vi "MegaAwesome_9_21_12b_JW.vi"() -> ()   [LabVIEW 2011]
uses:
  MegaAwesome_States.ctl
  <vilib>/Utility/inputDevices.llb/keyboardAcquire.vi
  <vilib>/Utility/file.llb/Read From Spreadsheet File (string).vi
  <vilib>/Utility/file.llb/Write To Spreadsheet File (string).vi
panel:
  out "ROI Descriptor out":T1 {"Contours"."Type" items=["No Selection", "Point", "Line", "Rectangle", "Oval", "Polygon", "Freehand Region", "Annulus", "Unused2", "Unused3", "Broken Line", "Freehand Line", "Rotated Rectangle"]}
  out "ROI Descriptor":T1 {"Contours"."Type" items=["No Selection", "Point", "Line", "Rectangle", "Oval", "Polygon", "Freehand Region", "Annulus", "Unused2", "Unused3", "Broken Line", "Freehand Line", "Rotated Rectangle"]}
  in  "Slider Min":dbl=5.0
  in  "Slider Max":dbl=5.0
  out "Opj X Axis":string
  out "X Axis Display Type":string
  in  "Index-Sat":dbl=5.0
  in  "Index-Lin":dbl=5.0
  in  "IndexLog-Lin":dbl=5.0
  in  "IndexLog-Sat":dbl=5.0 caption="Num Pts"
  out "Lin Id-Log Used":dbl[](array[numeric])
  out "Lin-Vg Array-Log Used":dbl[](array[numeric])
  in  "New: Comments":string
  out "Save Array":string[][](array[string])
  out "Folder Index":i32 caption="Length"
  out "Sat Id-Used":dbl[](array[numeric])
  out "Sat Vg Array-Used":dbl[](array[numeric])
  out "Vg Array-Log-Used":dbl[](array[numeric])
  out "Sat Id-Log-Used":dbl[](array[numeric])
  out "Lin Id-Used":dbl[](array[numeric])
  out "Lin-Vg Array-Used":dbl[](array[numeric])
  out "Lin Vd":dbl
  out "Recorded Prop":T2
  out "Current State":T3
  in  "Main Tab Control":T4(tab)
  in  "1) Transport":bool caption="2) Transport"
  in  "Image Analysis":bool caption="1) Image Analysis"
  in  "Transport\nFolder":path caption="Transport Folder"
  out "Transport\nFile":path=path "D:/UserData/Desktop/Jeremy/WFU/Research/Programs/VI mods/Image Not Found.png" caption="Transport File"
  in  "Image Folder":path
  out "Image File":path=path "D:/UserData/Desktop/Jeremy/WFU/Research/Programs/VI mods/Image Not Found.png"
  in  "Transfer File":path
  out "Transfer Folder":path
  out "Fabrication Prop":T5
  out "Distances":dbl[](array[numeric])
  in  "Zoom":i16(slide)=-3 scale=-5.0..5.0
  in  "Magnification":u16(ring) items=["5x", "10x", "20x", "50x", "80x"]
  in  "Undo Button":bool
  in  "Remove Button":bool
  in  "Transfer Plots":T6(tab)=enum."Saturation"
  in  "Lin-Trans Slider":dbl(slide) step=1.0 scale=-40.0..40.0 scale format="%#_1p"
  out "Sqrt-Lin":cluster{dbl[], dbl[]}[](graph)
  in  "Sat-Trans Slider":dbl(slide) step=1.0 scale=-40.0..40.0 scale format="%#_1p"
  out "Sqrt-Sat":cluster{dbl[], dbl[]}[](graph)
  out "Raw- Lin":cluster{dbl[], dbl[]}[](graph)
  out "Raw- Sat":cluster{dbl[], dbl[]}[](graph)
  in  "Log Plots":enum32{"Linear", "Saturation", "Transport"}(tab)=enum."Saturation"
  in  "Lin-Log Slider":dbl(slide) step=1.0 scale=-40.0..40.0 scale format="%#_1p"
  out "Log-Lin":cluster{dbl[], dbl[]}[](graph)
  in  "Sat-Log Slider":dbl(slide) step=1.0 scale=-40.0..40.0 scale format="%#_1p"
  out "Sat-Log":cluster{dbl[], dbl[]}[](graph)
  out "Transport":cluster{dbl[], dbl[]}[](graph)
  in  "Manual Controls":T7
  in  "File Controls":T8
  out "Date Recorded":string="Date Recorded" caption="Measured"
  out "Data Name:":string
  out "Image Name":string
  out "Index":string
  out "Date Created":string caption="Fabricated"
  in  "Comments:":string
  out "Rec: Length":dbl caption="Length" format="%#_3g"
  out "Rec: Width":dbl caption="Width" format="%#_4g"
  out "Rec: Dielectric (d)":dbl caption="Dielectric (d)" format="%#_3g"
  in  "New: Dielectric":dbl
  in  "New: Length":dbl
  in  "New: Width":dbl
  out "Rec: Temp":dbl caption="Sample Temp" format="%.1f"
  in  "New: Temp":dbl format="%.1f"
  out "Image Out":T9(plugin-control)
  in  "Num Pts":dbl=5.0
  in  "Num Pts Log":dbl=5.0 caption="Num Pts"
  out "Recorded Values Cluster":T10
  out "Calculated Values Cluster":T10 caption="Recorded Values Cluster"
  out "Re-Calculated Values Cluster":T10 caption="Recorded Values Cluster"
  in  "Independant Variable:":string(combo)="Length (um):"
  out "Image Preview":T9(plugin-control)
  out "Total Width":dbl
  in  "Room Temp":dbl=294.0
  in  "No Image\n File":path=path "\\\\acad1\\physics/Jurchescu-group/JW-PD/Mega Awesome/Image Not Found.png" caption="No Image File"
  in  "Origin Project File":path=path "\\\\acad1\\physics/Jurchescu-group/JW-PD/Group Library/Origin Project Files/DeviceData_8_10_12a_JW.opj"
  in  "No Transport\n File":path=path "\\\\acad1\\physics/Jurchescu-group/JW-PD/Mega Awesome/Image Not Found.png" caption="No Transport File"
  in  "Transport Style Controls":T11={"Transport Line Size"=1, "Transport Line Color"=16772608} {"Transport Line Size" items=["Extra Small", "Small", "Medium", "Large", "Extra Large"]}
  # "Transfer Location"
  # "What else would you like to view during your analysis?"
  # "Image Location"
  # "Transport Location"
  # "Recorded"
  # "Calculated"
  # "Re-Calculated"
  # "Manual"
  # "Used points display at y=0\nValues are wrong w/ slider"
  # "Slider\nDoesn't\nWork"
  # "Slider\nDoesn't\nWork"
  # "No new points displayed"
  # "Default File Choices"
  # "Default Analysis Values"
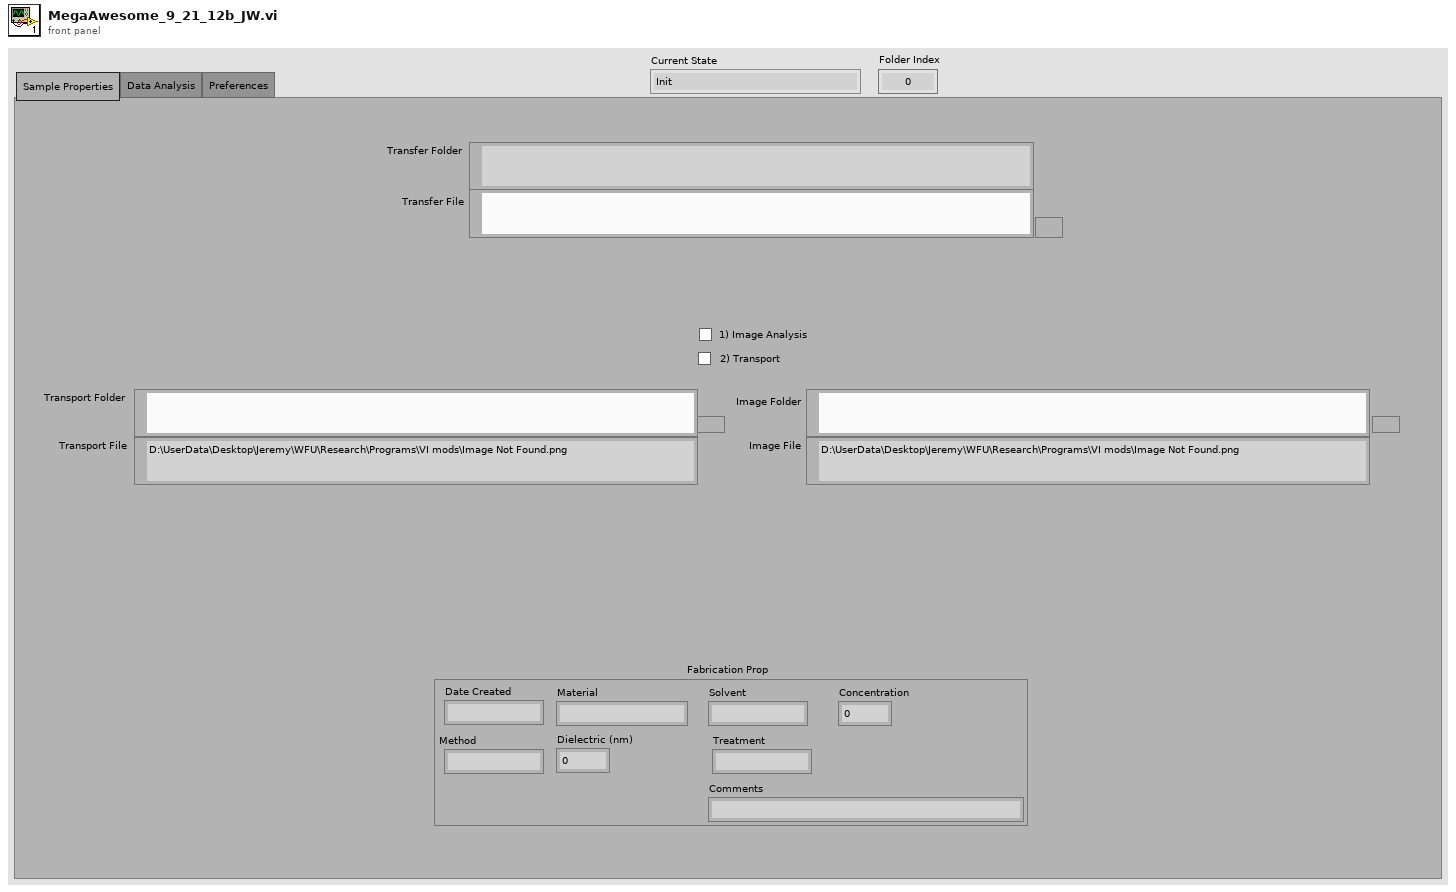
[diagram p1: front panel]
types:
  T1 = typedef "ROI Descriptor" = cluster{"Global Rectangle":i32[], "Contours":cluster{"ID":enum32{"External", "Internal"}, "Type":u32, "Coordinates":i32[]}[]}
  T2 = cluster{"Date Recorded":string, "Index":string, "Length":dbl, "Width":dbl, "Sample Temp":dbl}
  T3 = typedef "MegaAwesome_States.ctl" = enum16{"Init", "File Missing", "No Event", "Read Data", "Calculated Values", "Re-Calculated Values", "Next File", "Previous File", "Discard File", "Save", "Save Lines", "Export", "Exit"}
  T4 = enum32{"Sample Properties", "Data Analysis", "Preferences"}
  T5 = cluster{"Date Created":string, "Material":string, "Solvent":string, "Concentration":dbl, "Method":string, "Dielectric (nm)":dbl, "Treatment":string, "Comments":string}
  T6 = enum32{"Linear", "Saturation", "Raw-Linear", "Raw-Saturation"}
  T7 = cluster{"Manual-Temp":bool, "Manual-Width":bool, "Manuel-Length":bool, "Manuel-Dielectric":bool, "Manual Comments":bool}
  T8 = cluster{"Previous File":bool, "Discard ":bool, "Save Lines":bool, "Close":bool, "Next File ":bool, "Save":bool, "Save Next":bool, "Export":bool}
  T9 = typedef "IMAQ Image.ctl" = refnum<image>
  T10 = cluster{"Mobility-Sat":dbl, "Moblitity-Lin":dbl, "On/Off":dbl, "Off Current":dbl, "Vt-Sat":dbl, "STS":dbl, "Trap Density-VT":dbl, "Trap Density-STS":dbl}
  T11 = cluster{"Transport Line Size":u16, "Transport Line Color":u32}
  T12 = typedef "LVBoundsTypeDef.ctl" = cluster{"Width":u32, "Height":u32}
  T13 = cluster{"Global Rectangle":i32[], "Contours":cluster{"Contour Type":u32, "ROI Type":u32, "Points":i32[]}[]}
  T14 = cluster{"Contour Type":u32, "ROI Type":u32, "Points":i32[]}[]
  T15 = cluster{i32[], cluster{"Contour Type":u32, "ROI Type":u32, "Points":i32[]}[]}
  T16 = enum16{"0", "1", "2", "3", "4", "5", "6", "7", "8", "9", "A", "B", "C", "D", "E", "F", "G", "H", "I", "J", "K", "L", "M", "N", "O", "P", "Q", "R", "S", "T", "U", "V", "W", "X", "Y", "Z", "F1", "F2", "F3", "F4", "F5", "F6", "F7", "F8", "F9", "F10", "F11", "F12", "F13", "F14", "F15", "ADD", "BACK", "BACKSLASH", "CAPITAL", "COMMA", "DECIMAL", "DELETE", "DIVIDE", "DOWN", "END", "EQUALS", "ESCAPE", "GRAVE (`)", "HOME", "INSERT", "LBRACKET", "LCONTROL", "LEFT", "L ALT", "LSHIFT", "LWIN", "MINUS", "MULTIPLY", "NEXT", "NUMLOCK", "NUMPAD_0", "NUMPAD_1", "NUMPAD_2", "NUMPAD_3", "NUMPAD_4", "NUMPAD_5", "NUMPAD_6", "NUMPAD_7", "NUMPAD_8", "NUMPAD_9", "PAUSE", "PERIOD", "PRIOR (PG UP)", "RBRACKET", "RCONTROL", "RETURN", "RIGHT", "R ALT", "RSHIFT", "RWIN", "SCROLL", "SEMICOLON", "SLASH", "SPACE", "SUBTRACT", "TAB", "UP", "ENTER (num pad)", "' (quote)"}[]
  T17 = enum16{"0", "1", "2", "3", "4", "5", "6", "7", "8", "9", "A", "B", "C", "D", "E", "F", "G", "H", "I", "J", "K", "L", "M", "N", "O", "P", "Q", "R", "S", "T", "U", "V", "W", "X", "Y", "Z", "F1", "F2", "F3", "F4", "F5", "F6", "F7", "F8", "F9", "F10", "F11", "F12", "F13", "F14", "F15", "ADD", "BACK", "BACKSLASH", "CAPITAL", "COMMA", "DECIMAL", "DELETE", "DIVIDE", "DOWN", "END", "EQUALS", "ESCAPE", "GRAVE (`)", "HOME", "INSERT", "LBRACKET", "LCONTROL", "LEFT", "L ALT", "LSHIFT", "LWIN", "MINUS", "MULTIPLY", "NEXT", "NUMLOCK", "NUMPAD_0", "NUMPAD_1", "NUMPAD_2", "NUMPAD_3", "NUMPAD_4", "NUMPAD_5", "NUMPAD_6", "NUMPAD_7", "NUMPAD_8", "NUMPAD_9", "PAUSE", "PERIOD", "PRIOR (PG UP)", "RBRACKET", "RCONTROL", "RETURN", "RIGHT", "R ALT", "RSHIFT", "RWIN", "SCROLL", "SEMICOLON", "SLASH", "SPACE", "SUBTRACT", "TAB", "UP", "ENTER (num pad)", "' (quote)"}
  T18 = cluster{string, sgl, bool, bool, bool, bool, bool, bool, i32}
  T19 = cluster{i32, cluster{string, sgl, bool, bool, bool, bool, bool, bool, i32}, i32, i32}
  T20 = cluster{"Contour Type":u32, "ROI Type":u32, "Points":i32[]}
  T21 = cluster{"Points[0]":i32, "Points[1]":i32, "Points[2]":i32, "Points[3]":i32, "Points[4]":i32, "Points[5]":i32, "Points[6]":i32, "Points[7]":i32, "Points[8]":i32}
  T22 = cluster{"[0]":cluster{dbl[], dbl[]}, "[1]":cluster{dbl[], dbl[]}, "[2]":cluster{dbl[], dbl[]}, "[3]":cluster{dbl[], dbl[]}, "[4]":cluster{dbl[], dbl[]}, "[5]":cluster{dbl[], dbl[]}, "[6]":cluster{dbl[], dbl[]}, "[7]":cluster{dbl[], dbl[]}, "[8]":cluster{dbl[], dbl[]}}
  T23 = cluster{"Sat Vg Used":dbl[], "Sat Sqrt(Id) Used ":dbl[], "Lin Vg Used":dbl[], "Lin Sqrt(Id) Used":dbl[], "Index-Lin":dbl, "Index-Sat":dbl}
  T24 = cluster{"Raw Sat":cluster{dbl[], dbl[]}[], "Sqrt Sat":cluster{dbl[], dbl[]}[], "Log Sat":cluster{dbl[], dbl[]}[], "Raw Lin":cluster{dbl[], dbl[]}[], "Sqrt Lin":cluster{dbl[], dbl[]}[], "Log Lin":cluster{dbl[], dbl[]}[]}
  T25 = cluster{"Mobility-Sat":dbl, "Vt-Sat":dbl, "Mobility-Lin":dbl, "Vt-Lin":dbl, "Off I-Sat":dbl, "On/Off I-Sat":dbl}
  T26 = cluster{"Sat Vg Used":dbl[], "Sat Log(Id) Used":dbl[], "Lin Vg Used":dbl[], "Lin Log(Id) Used":dbl[], "STS Index-Sat":dbl, "STS Index-Lin":dbl}
  T27 = cluster{"Independant  Variable Indicator":string, "Parameter String Indicator":string}
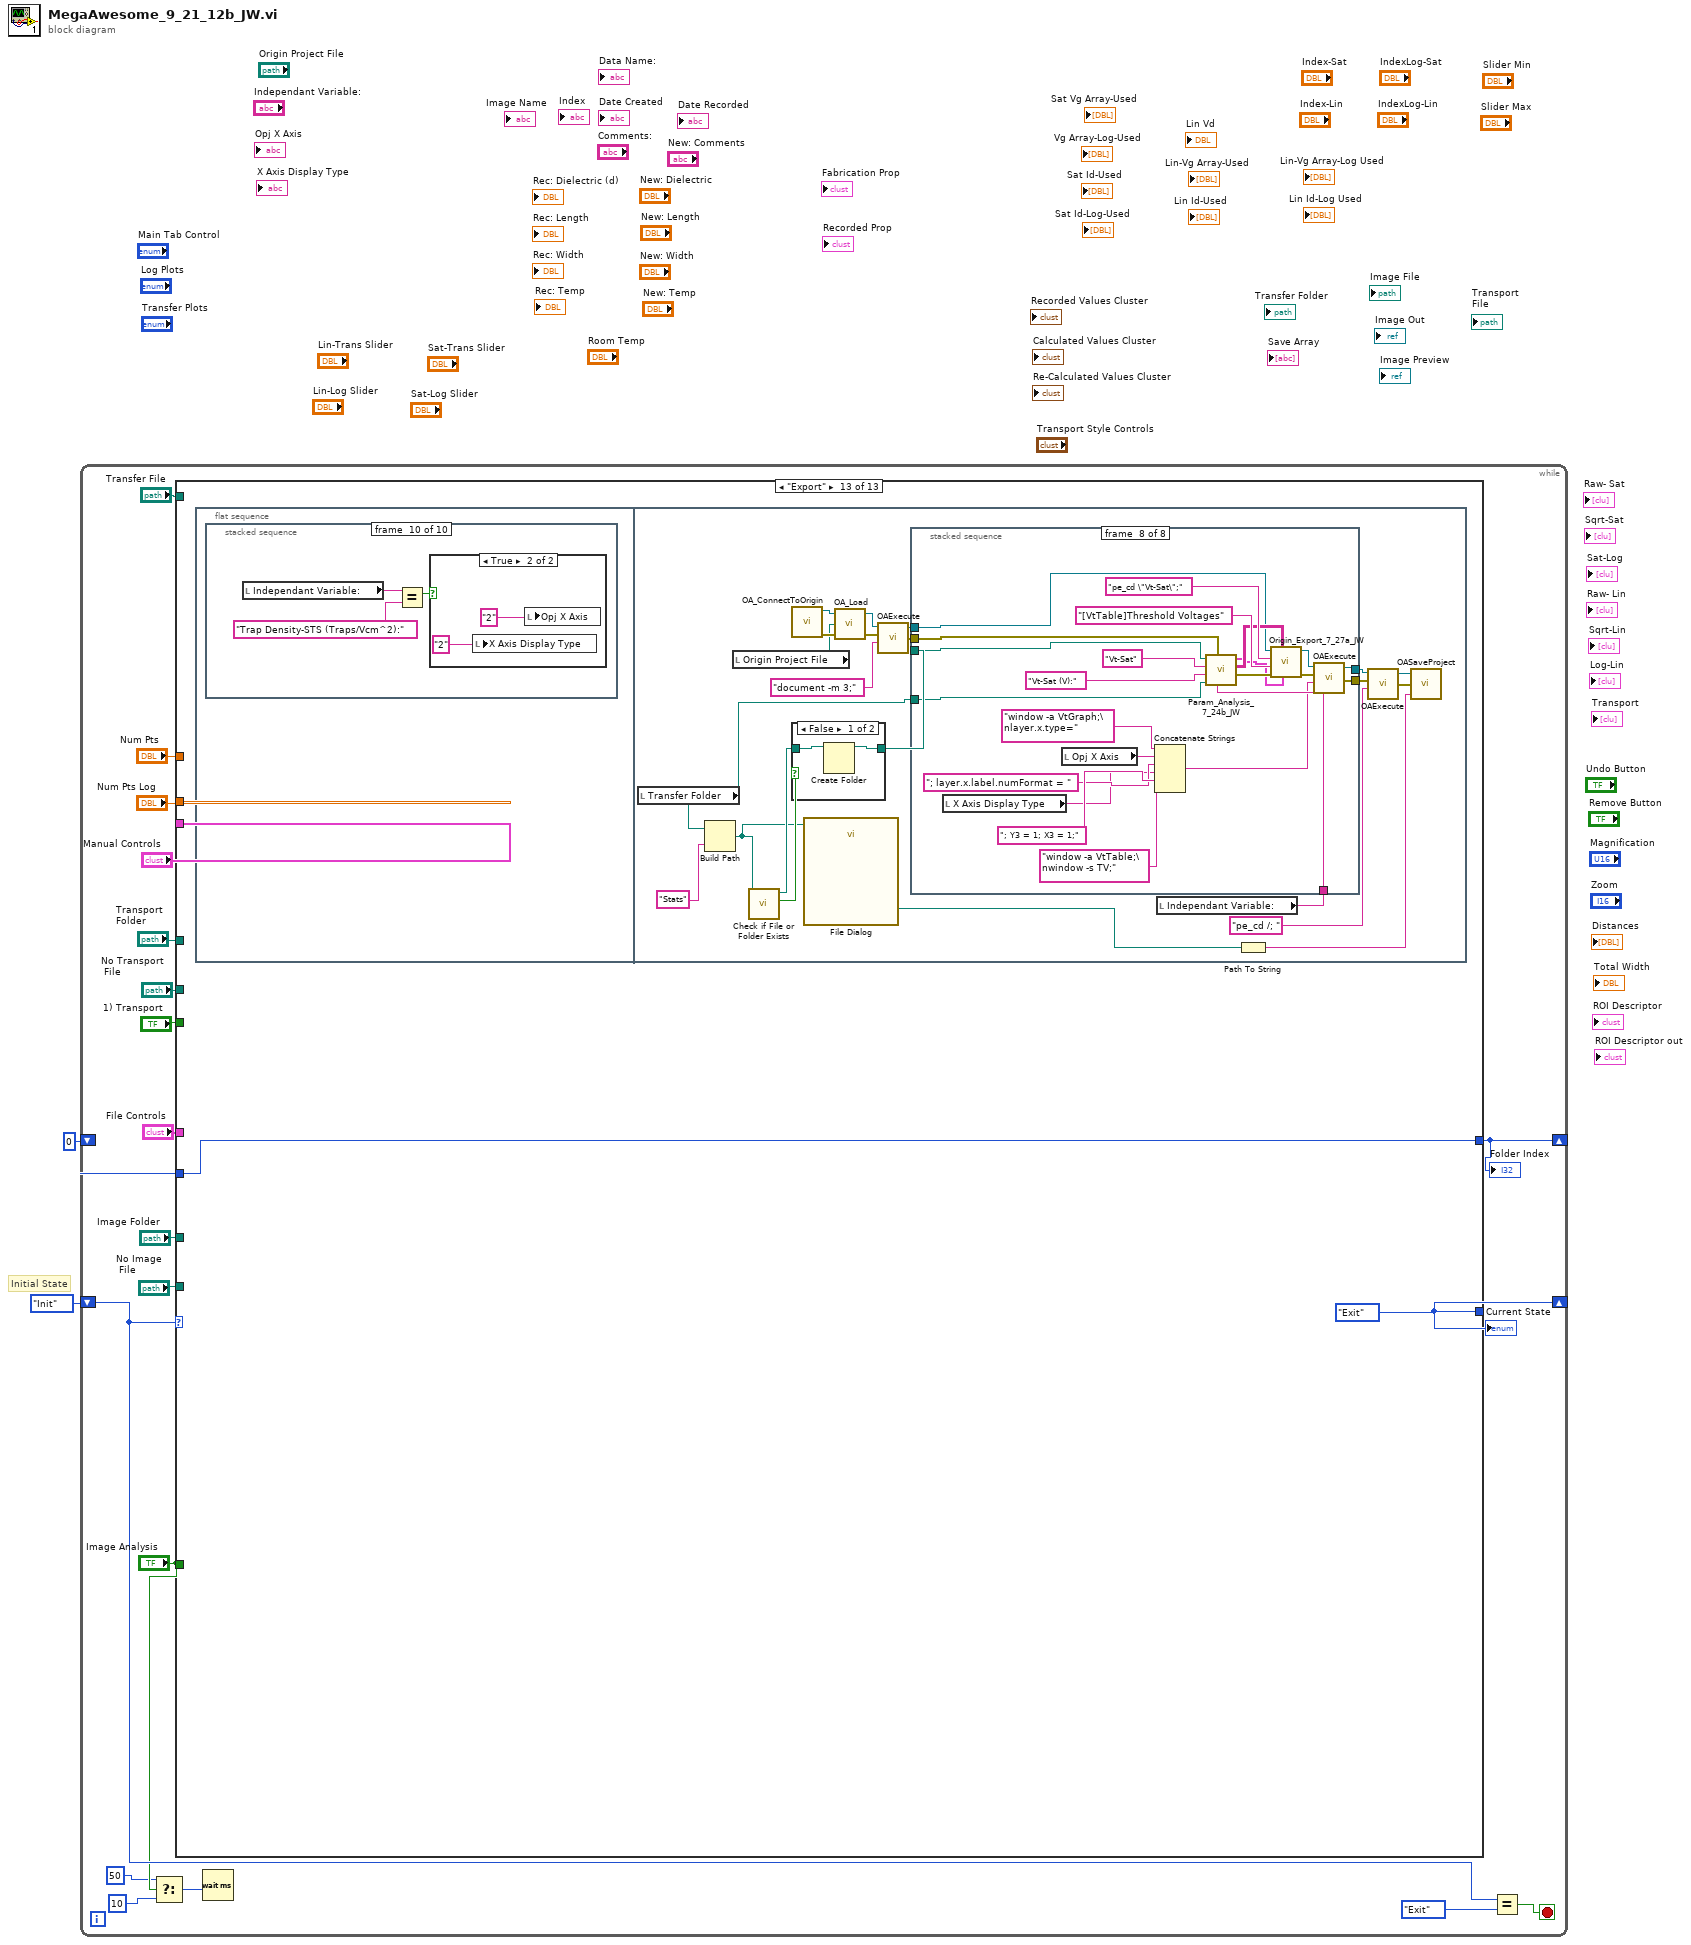
[diagram p0: block diagram]
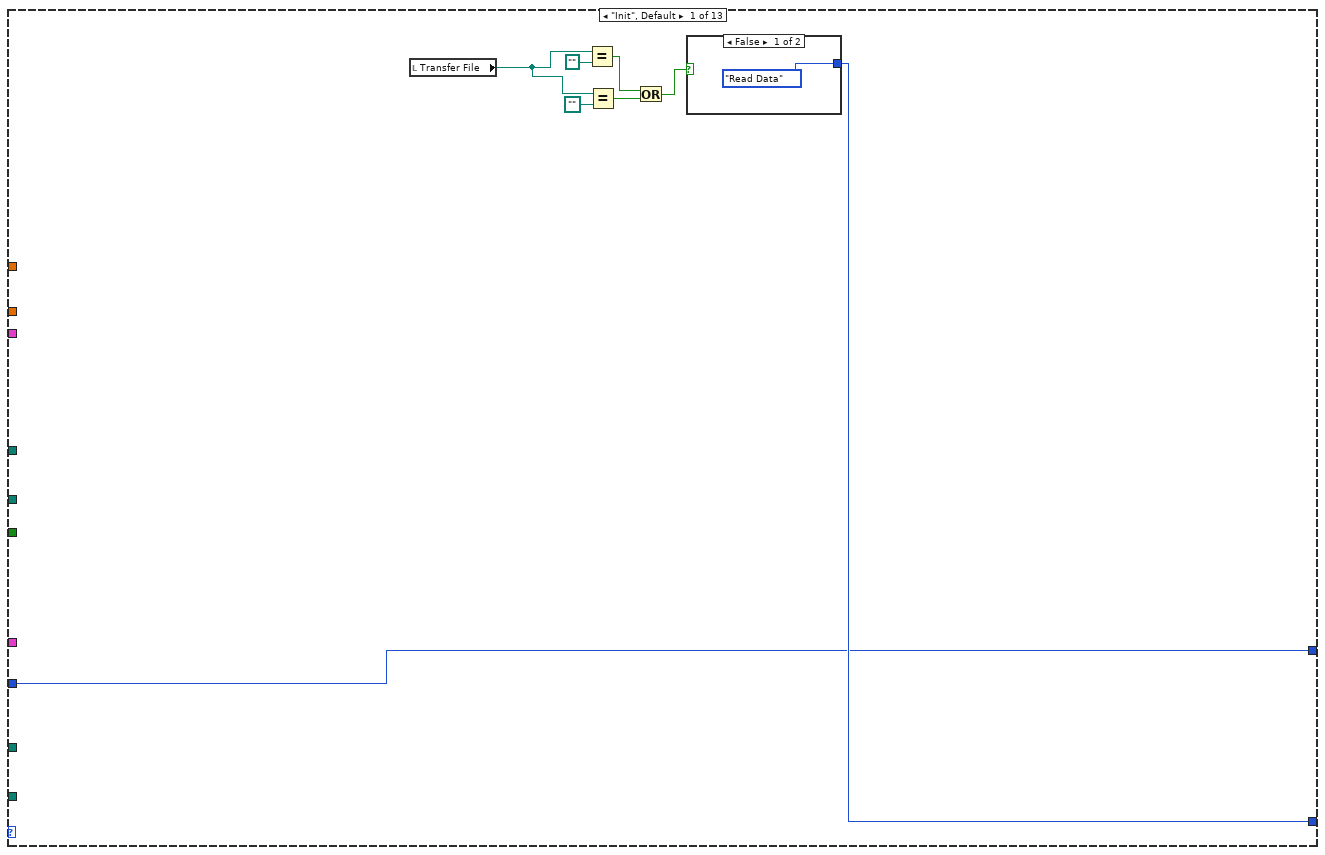
[diagram p2: hidden frame]
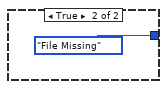
[diagram p3: hidden frame]
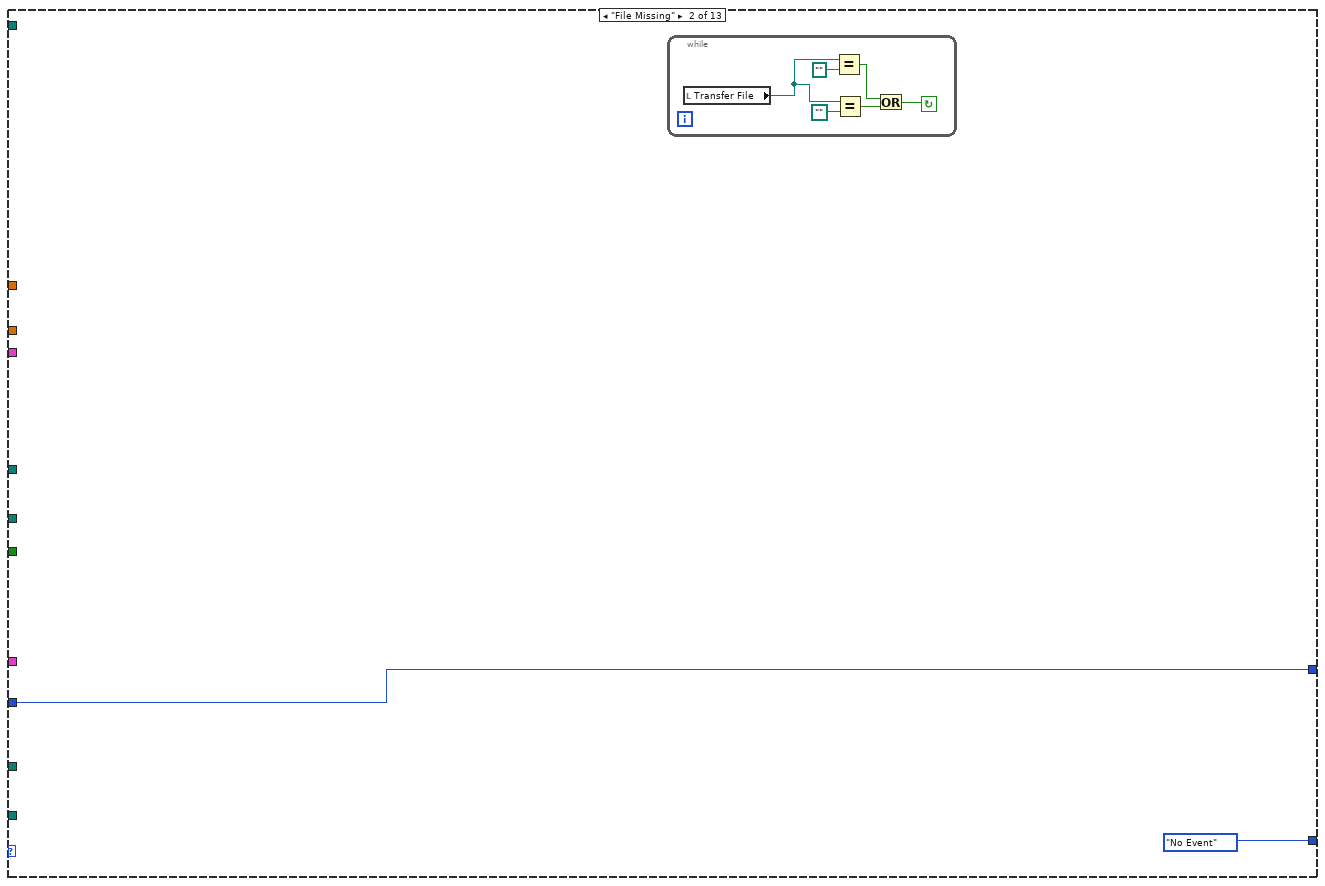
[diagram p4: hidden frame]
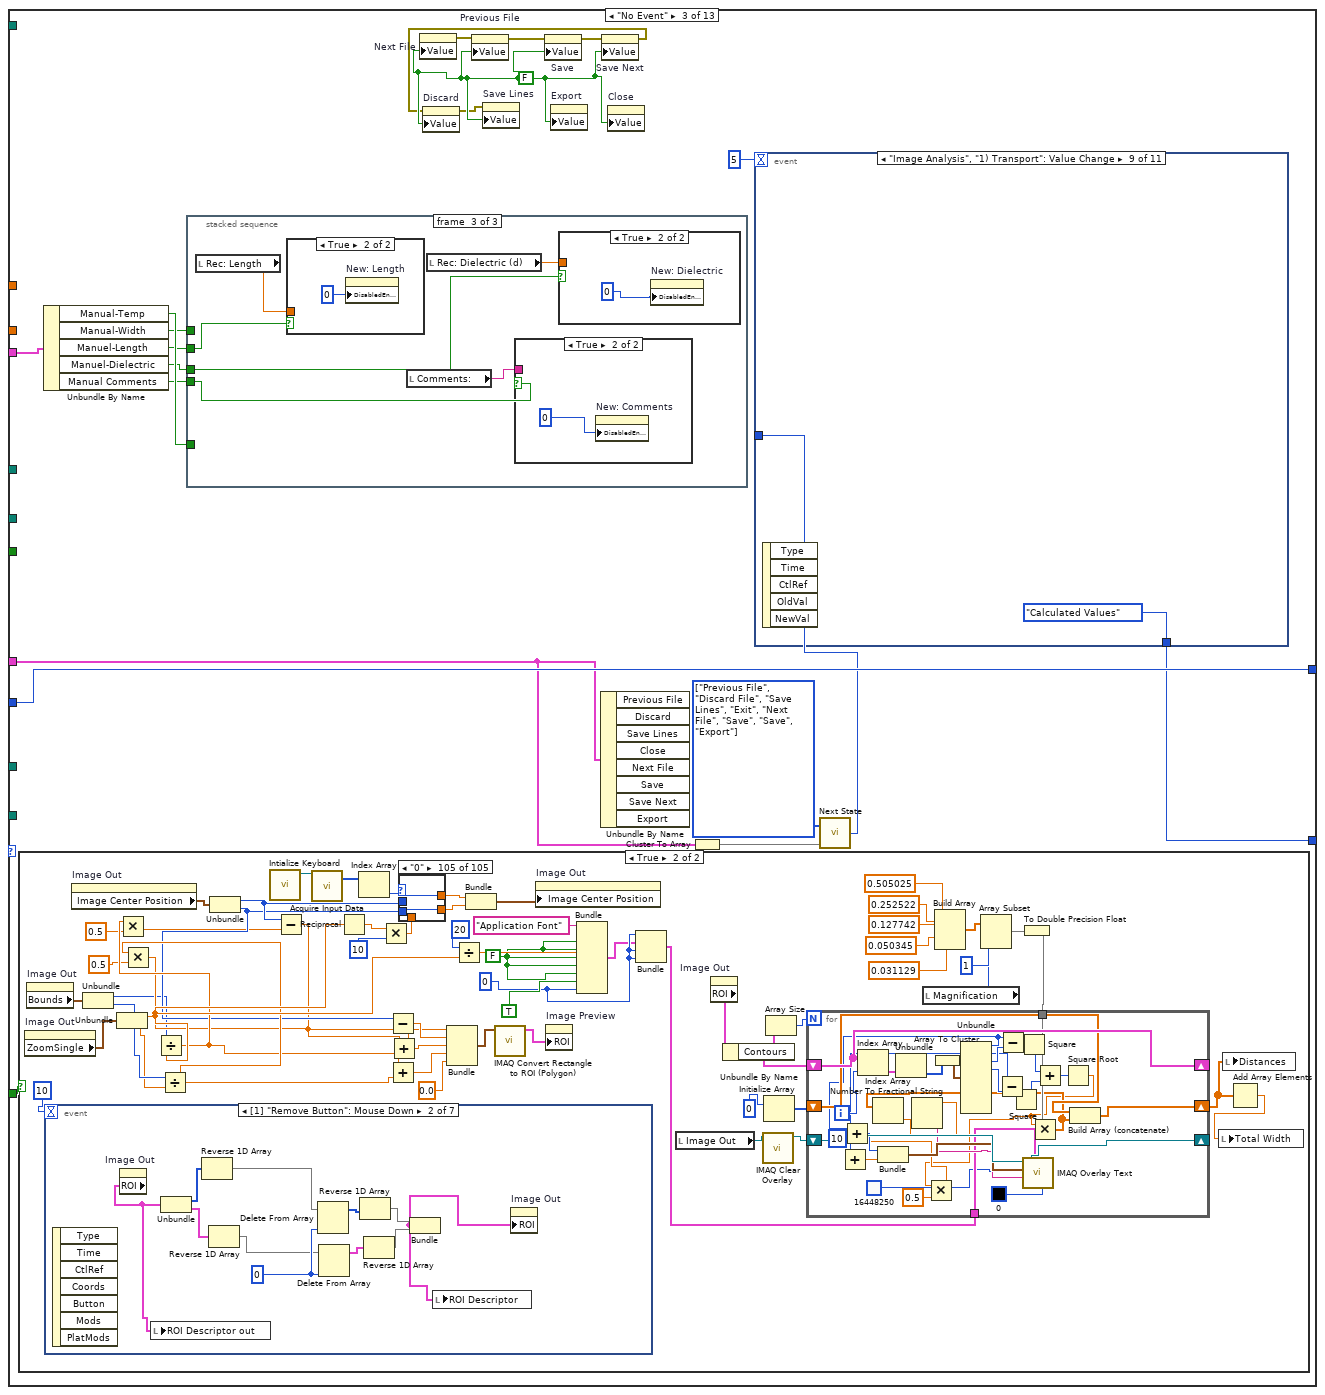
[diagram p5: hidden frame]
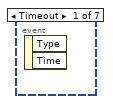
[diagram p7: hidden frame]
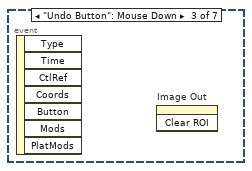
[diagram p8: hidden frame]
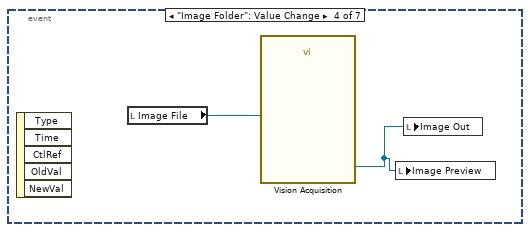
[diagram p9: hidden frame]
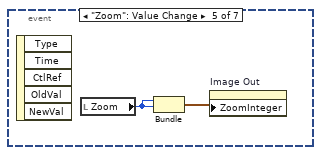
[diagram p10: hidden frame]
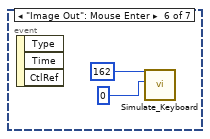
[diagram p11: hidden frame]
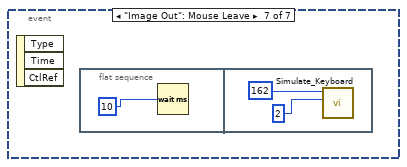
[diagram p12: hidden frame]
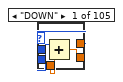
[diagram p13: hidden frame]
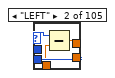
[diagram p14: hidden frame]
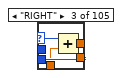
[diagram p15: hidden frame]
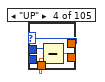
[diagram p16: hidden frame]
diagram:
  # "Initial State"
  n1 = while {
    shift-right: [w19] -> _
    shift-left: MegaAwesome_States."Init" -> [w21]
    shift-right: [w12] -> _
    shift-left: 0 -> [w13]
    stop <- w22 stop-if-true
    n2 = Select(t=50, s="Image Analysis", f=10) -> (s? t:f=w6:i32)
    n3 = case shown="\"Export\"" w21 {
      tunnel: [w24 MegaAwesome_States."No Event" w50 MegaAwesome_States."Calculated Values" MegaAwesome_States."Re-Calculated Values" MegaAwesome_States."No Event" MegaAwesome_States."Read Data" MegaAwesome_States."Read Data" MegaAwesome_States."No Event" w697 MegaAwesome_States."No Event" MegaAwesome_States."No Event" MegaAwesome_States."Exit"] -> w19
      tunnel: "Transfer File" -> [_ _ _ w525 w559 _ w666 w678 _ w702 _ _ _]
      tunnel: "Num Pts" -> [_ _ _ _ w583 _ _ _ _ _ _ _ _]
      tunnel: "Num Pts Log" -> [_ _ _ _ w582 _ _ _ _ _ _ _ _]
      tunnel: "Image Folder" -> [_ _ _ _ w579 _ _ _ _ _ _ _ _]
      tunnel: "No Image\n File" -> [_ _ _ _ w578 _ _ _ _ _ _ _ _]
      tunnel: [w23 w33 w58 w519 w577 w626 w651 w676 w694 w703 w1218 w1221 w1222] -> w12
      tunnel: w13 -> [w23 w33 w58 _ w577 w626 w652 w677 w694 w703 w1218 w1221 w1222]
      tunnel: "Manual Controls" -> [_ _ w52 _ _ _ _ _ _ w701 _ _ _]
      tunnel: "File Controls" -> [_ _ w48 _ _ _ _ _ _ w696 _ _ _]
      tunnel: "1) Transport" -> [_ _ _ _ w549 _ _ _ _ _ _ _ _]
      tunnel: "Image Analysis" -> [_ _ w41 _ w548 _ _ _ _ _ _ _ _]
      tunnel: "Transport\nFolder" -> [_ _ _ _ w547 _ _ _ _ _ _ _ _]
      tunnel: "No Transport\n File" -> [_ _ _ _ w546 _ _ _ _ _ _ _ _]
      frame "Init", Default {
        n4 = local read "Transfer File"() -> (w25:path)
        n5 = Equal?(x=w25, y=path "") -> (x = y?=w28:bool)
        n6 = Equal?(x=w25, y=path "") -> (x = y?=w27:bool)
        n7 = Or(x=w28, y=w27) -> (x .or. y?=w30:bool)
        n8 = case shown="False" w30 {
          tunnel: [MegaAwesome_States."Read Data" MegaAwesome_States."File Missing"] -> w24
          frame False {
          }
          frame True {
          }
        }
      }
      frame "File Missing" {
        n9 = while {
          stop <- w35 continue-if-true
          n10 = local read "Transfer File"() -> (w36:path)
          n11 = Equal?(x=w36, y=path "") -> (x = y?=w38:bool)
          n12 = Equal?(x=w36, y=path "") -> (x = y?=w39:bool)
          n13 = Or(x=w38, y=w39) -> (x .or. y?=w35:bool)
        }
      }
      frame "No Event" {
        w47 = FALSE
        w60 = T3[] [enum."Previous File", enum."Discard File", enum."Save Lines", enum."Exit", enum."Next File", enum."Save", enum."Save", enum."Export"] items=["Init", "File Missing", "No Event", "Read Data", "Calculated Values", "Re-Calculated Values", "Next File", "Previous File", "Discard File", "Save", "Save Lines", "Export", "Exit"]
        n14 = case shown="True" w41 {
          frame False {
          }
          frame True {
            w110 = FALSE
            w112 = 0
            n15 = property on="Image Out" class="ImageControl"() -> ("ZoomSingle"=w95:cluster{"X":sgl, "Y":sgl})  [unwired: 2 in, 2 out]
            n16 = property on="Image Out" class="ImageControl"() -> ("Bounds"=w94:T12)  [unwired: 2 in, 2 out]
            n17 = event shown="[1] \"Remove Button\": Mouse Down" {
              selector: _ -> [_ _ _ _ _ _ _]
              dyn-events: _ -> [_ _ _ _ _ _ _]
              timeout: 10 -> [_ _ _ _ _ _ _]
              event Timeout {
                n18 = event-data() -> ()  [unwired: 1 in, 2 out]
              }
              event "Remove Button": Mouse Down {
                w130 = 0
                n19 = event-data() -> ()  [unwired: 1 in, 7 out]
                n20 = property on="Image Out" class="ImageControl"() -> ("ROI"=w120:T13)  [unwired: 2 in, 2 out]
                n21 = local write "ROI Descriptor out"(w120) -> ()
                n22 = Unbundle(w120) -> ("Global Rectangle"=w129:i32[], "Contours"=w127:T14)
                n23 = Reverse 1D Array(array=w129) -> (reversed array=w128:i32[])
                n24 = Reverse 1D Array(array=w127) -> (reversed array=w126:T14)
                n25 = Delete From Array(array=w128, index=w130) -> (array with subset deleted=w125:i32[])  [unwired: 1 in, 1 out]
                n26 = Delete From Array(array=w126, index=w130) -> (array with subset deleted=w124:T14)  [unwired: 1 in, 1 out]
                n27 = Reverse 1D Array(array=w125) -> (reversed array=w123:i32[])
                n28 = Reverse 1D Array(array=w124) -> (reversed array=w122:T14)
                n29 = Bundle(w123, w122) -> (w121:T15)  [unwired: 1 in]
                n30 = local write "ROI Descriptor"(w121) -> ()
                n31 = property on="Image Out" class="ImageControl"("ROI"=w121) -> ()  [unwired: 2 in, 2 out]
              }
              event "Undo Button": Mouse Down {
                n32 = event-data() -> ()  [unwired: 1 in, 7 out]
                n33 = invoke on="Image Out" class="ImageControl" method="Clear ROI"() -> ()  [unwired: 3 in, 3 out]
              }
              event "Image Folder": Value Change {
                n34 = event-data() -> ()  [unwired: 1 in, 5 out]
                n35 = local read "Image File"() -> (w132:path)
                n36 = call "Vision Acquisition"("Image Path"=w132) -> ("Image Out"=w131:T9)  [unwired: 25 in, 1 out]
                n37 = local write "Image Preview"(w131) -> ()
                n38 = local write "Image Out"(w131) -> ()
              }
              event "Zoom": Value Change {
                n39 = event-data() -> ()  [unwired: 1 in, 5 out]
                n40 = local read "Zoom"() -> (w133:i16)
                n41 = Bundle("Zoom"=w133, "Zoom"=w133) -> (w134:cluster{"Zoom":i16, "Zoom":i16})  [unwired: 1 in]
                n42 = property on="Image Out" class="ImageControl"("ZoomInteger"=w134) -> ()  [unwired: 2 in, 2 out]
              }
              event "Image Out": Mouse Enter {
                n43 = event-data() -> ()  [unwired: 1 in, 3 out]
                n44 = call "Simulate_Keyboard.vi"("Action"=0, "Virtual Key"=162) -> ()  [unwired: 7 in, 1 out]
              }
              event "Image Out": Mouse Leave {
                n45 = event-data() -> ()  [unwired: 1 in, 3 out]
                n46 = flat-sequence {
                  frame #0 {
                    n47 = Wait (ms)(milliseconds to wait=10) -> ()  [unwired: 1 out]
                  }
                  frame #1 {
                    n48 = call "Simulate_Keyboard.vi"("Action"=2, "Virtual Key"=162) -> ()  [unwired: 7 in, 1 out]
                  }
                }
              }
            }
            n49 = property on="Image Out" class="ImageControl"() -> ("Image Center Position"=w88:cluster{"X":u32, "Y":u32})  [unwired: 2 in, 2 out]
            n50 = Unbundle(w94) -> ("Width"=w97:u32, "Height"=w98:u32)
            n51 = Unbundle(w95) -> ("X"=w117:sgl, "Y"=w96:sgl)
            n52 = Divide(x=w97, y=w117) -> (x/y=w107:sgl)
            n53 = Multiply(x=w107, y=0.5) -> (x*y=w101:dbl)
            n54 = Divide(x=w98, y=w96) -> (x/y=w108:sgl)
            n55 = Multiply(x=w108, y=0.5) -> (x*y=w102:dbl)
            n56 = Unbundle(w88) -> ("X"=w106:u32, "Y"=w105:u32)
            n57 = call <vilib>:"Intialize Keyboard.vi"() -> ("device ID"=w85:refnum<k1>)  [unwired: 10 in, 1 out]
            n58 = Subtract(x=w106, y=w101) -> (x-y=w103:dbl)
            n59 = call-poly <vilib>:"Acquire Input Data.vi"("device ID"=w85) -> ("keys pressed"=w86:T16)  [unwired: 16 in, 2 out]
            n60 = Reciprocal(x=w117) -> (1/x=w118:sgl)
            n61 = Index Array(array=w86) -> (element=w82:T17)  [unwired: 1 in]
            n62 = Multiply(x=w118, y=10) -> (x*y=w116:sgl)
            n63 = Subtract(x=w105, y=w102) -> (x-y=w104:dbl)
            n64 = Add(x=w104, y=w108) -> (x+y=w90:dbl)
            n65 = Add(x=w103, y=w107) -> (x+y=w89:dbl)
            n66 = case shown="\"0\"" w82 {
              tunnel: w106 -> [w173 w179 w183 w185 w189 w191 w193 w195 w197 w199 w201 w203 w205 w207 w209 w211 w213 w215 w217 w219 w221 w223 w225 w227 w229 w231 w233 w235 w237 w239 w241 w243 w245 w247 w249 w251 w253 w255 w257 w259 w261 w263 w265 w267 w269 w271 w273 w275 w277 w279 w281 w283 w285 w287 w289 w291 w293 w295 w297 w299 w301 w303 w305 w307 w309 w311 w313 w315 w317 w319 w321 w323 w325 w327 w329 w331 w333 w335 w337 w339 w341 w343 w345 w347 w349 w351 w353 w355 w357 w359 w361 w363 w365 w367 w369 w371 w373 w375 w377 w379 w381 w383 w385 w387 w389]
              tunnel: [w173 w178 w182 w185 w189 w191 w193 w195 w197 w199 w201 w203 w205 w207 w209 w211 w213 w215 w217 w219 w221 w223 w225 w227 w229 w231 w233 w235 w237 w239 w241 w243 w245 w247 w249 w251 w253 w255 w257 w259 w261 w263 w265 w267 w269 w271 w273 w275 w277 w279 w281 w283 w285 w287 w289 w291 w293 w295 w297 w299 w301 w303 w305 w307 w309 w311 w313 w315 w317 w319 w321 w323 w325 w327 w329 w331 w333 w335 w337 w339 w341 w343 w345 w347 w349 w351 w353 w355 w357 w359 w361 w363 w365 w367 w369 w371 w373 w375 w377 w379 w381 w383 w385 w387 w389] -> w83
              tunnel: w105 -> [w175 w177 w181 w187 w188 w190 w192 w194 w196 w198 w200 w202 w204 w206 w208 w210 w212 w214 w216 w218 w220 w222 w224 w226 w228 w230 w232 w234 w236 w238 w240 w242 w244 w246 w248 w250 w252 w254 w256 w258 w260 w262 w264 w266 w268 w270 w272 w274 w276 w278 w280 w282 w284 w286 w288 w290 w292 w294 w296 w298 w300 w302 w304 w306 w308 w310 w312 w314 w316 w318 w320 w322 w324 w326 w328 w330 w332 w334 w336 w338 w340 w342 w344 w346 w348 w350 w352 w354 w356 w358 w360 w362 w364 w366 w368 w370 w372 w374 w376 w378 w380 w382 w384 w386 w388]
              tunnel: [w174 w177 w181 w186 w188 w190 w192 w194 w196 w198 w200 w202 w204 w206 w208 w210 w212 w214 w216 w218 w220 w222 w224 w226 w228 w230 w232 w234 w236 w238 w240 w242 w244 w246 w248 w250 w252 w254 w256 w258 w260 w262 w264 w266 w268 w270 w272 w274 w276 w278 w280 w282 w284 w286 w288 w290 w292 w294 w296 w298 w300 w302 w304 w306 w308 w310 w312 w314 w316 w318 w320 w322 w324 w326 w328 w330 w332 w334 w336 w338 w340 w342 w344 w346 w348 w350 w352 w354 w356 w358 w360 w362 w364 w366 w368 w370 w372 w374 w376 w378 w380 w382 w384 w386 w388] -> w84
              tunnel: w116 -> [w172 w176 w180 w184 _ _ _ _ _ _ _ _ _ _ _ _ _ _ _ _ _ _ _ _ _ _ _ _ _ _ _ _ _ _ _ _ _ _ _ _ _ _ _ _ _ _ _ _ _ _ _ _ _ _ _ _ _ _ _ _ _ _ _ _ _ _ _ _ _ _ _ _ _ _ _ _ _ _ _ _ _ _ _ _ _ _ _ _ _ _ _ _ _ _ _ _ _ _ _ _ _ _ _ _ _]
              frame "DOWN" {
                n67 = Add(x=w175, y=w172) -> (x+y=w174:sgl)
              }
              frame "LEFT" {
                n68 = Subtract(x=w179, y=w176) -> (x-y=w178:sgl)
              }
              frame "RIGHT" {
                n69 = Add(x=w183, y=w180) -> (x+y=w182:sgl)
              }
              frame "UP" {
                n70 = Subtract(x=w187, y=w184) -> (x-y=w186:sgl)
              }
              frame "ENTER (num pad)" {
              }
              frame "' (quote)" {
              }
              frame "END" {
              }
              frame "EQUALS" {
              }
              frame "ESCAPE" {
              }
              frame "GRAVE (`)" {
              }
              frame "HOME" {
              }
              frame "INSERT" {
              }
              frame "LBRACKET" {
              }
              frame "LCONTROL" {
              }
              frame "L ALT" {
              }
              frame "LSHIFT" {
              }
              frame "LWIN" {
              }
              frame "MINUS" {
              }
              frame "MULTIPLY" {
              }
              frame "NEXT" {
              }
              frame "NUMLOCK" {
              }
              frame "NUMPAD_0" {
              }
              frame "NUMPAD_1" {
              }
              frame "NUMPAD_2" {
              }
              frame "NUMPAD_3" {
              }
              frame "NUMPAD_4" {
              }
              frame "NUMPAD_5" {
              }
              frame "NUMPAD_6" {
              }
              frame "NUMPAD_7" {
              }
              frame "NUMPAD_8" {
              }
              frame "NUMPAD_9" {
              }
              frame "PAUSE" {
              }
              frame "PERIOD" {
              }
              frame "PRIOR (PG UP)" {
              }
              frame "RBRACKET" {
              }
              frame "RCONTROL" {
              }
              frame "RETURN" {
              }
              frame "R ALT" {
              }
              frame "RSHIFT" {
              }
              frame "RWIN" {
              }
              frame "SCROLL" {
              }
              frame "SEMICOLON" {
              }
              frame "SLASH" {
              }
              frame "SPACE" {
              }
              frame "SUBTRACT" {
              }
              frame "TAB" {
              }
              frame "DIVIDE" {
              }
              frame "DELETE" {
              }
              frame "DECIMAL" {
              }
              frame "COMMA" {
              }
              frame "CAPITAL" {
              }
              frame "BACKSLASH" {
              }
              frame "BACK" {
              }
              frame "ADD" {
              }
              frame "F15" {
              }
              frame "F14" {
              }
              frame "F13" {
              }
              frame "F12" {
              }
              frame "F11" {
              }
              frame "F10" {
              }
              frame "F9" {
              }
              frame "F8" {
              }
              frame "F7" {
              }
              frame "F6" {
              }
              frame "F5" {
              }
              frame "F4" {
              }
              frame "F3" {
              }
              frame "F2" {
              }
              frame "F1" {
              }
              frame "Z" {
              }
              frame "Y" {
              }
              frame "X" {
              }
              frame "W" {
              }
              frame "V" {
              }
              frame "U" {
              }
              frame "T" {
              }
              frame "S" {
              }
              frame "R" {
              }
              frame "Q" {
              }
              frame "P" {
              }
              frame "O" {
              }
              frame "N" {
              }
              frame "M" {
              }
              frame "L" {
              }
              frame "K" {
              }
              frame "J" {
              }
              frame "I" {
              }
              frame "H" {
              }
              frame "G" {
              }
              frame "F" {
              }
              frame "E" {
              }
              frame "D" {
              }
              frame "C" {
              }
              frame "B" {
              }
              frame "A" {
              }
              frame "9" {
              }
              frame "8" {
              }
              frame "7" {
              }
              frame "6" {
              }
              frame "5" {
              }
              frame "4" {
              }
              frame "3" {
              }
              frame "2" {
              }
              frame "1" {
              }
              frame "0" {
              }
            }
            n71 = Bundle(w103, w104, w89, w90, 0.0) -> (w91:cluster{dbl, dbl, dbl, dbl, dbl})  [unwired: 1 in]
            n72 = Divide(x=20, y=w117) -> (x/y=w114:sgl)
            n73 = Bundle("X"=w83, "Y"=w84) -> (w87:cluster{"X":sgl, "Y":sgl})  [unwired: 1 in]
            n74 = call "IMAQ Convert Rectangle to ROI (Polygon)"("Rectangle"=w91) -> ("ROI Descriptor"=w93:T1)  [unwired: 7 in, 2 out]
            n75 = property on="Image Out" class="ImageControl"("Image Center Position"=w87) -> ()  [unwired: 2 in, 2 out]
            n76 = property on="Image Preview" class="ImageControl"("ROI"=w93) -> ()  [unwired: 2 in, 2 out]
            n77 = Bundle("Application Font", w114, w110, w110, w110, w110, w110, TRUE, w112) -> (w109:T18)  [unwired: 1 in]
            n78 = Bundle(w112, w109, w112, w112) -> (w63:T19)  [unwired: 1 in]
            n79 = local read "Image Out"() -> (w62:T9)
            n80 = property on="Image Out" class="ImageControl"() -> ("ROI"=w66:T13)  [unwired: 2 in, 2 out]
            n81 = Unbundle By Name(w66) -> ("Contours"=w67:T14)
            n82 = call "IMAQ Clear Overlay"("Image"=w62) -> ("Image Out"=w81:T9)  [unwired: 9 in, 1 out]
            n83 = Initialize Array(0) -> (w69:i32[])  [unwired: 1 in]
            n84 = Array Size(array=w67) -> (size(s)=w68:i32)
            n85 = local read "Magnification"() -> (w77:u16)
            n86 = Build Array(0.505025, 0.252522, 0.127742, 0.050345, 0.031129) -> (w76:dbl[])
            n87 = Array Subset(array=w76, index=w77, length=1) -> (w79:dbl[])
            n88 = To Double Precision Float(number=w79) -> (double precision float=w80:dbl[])
            n89 = for {
              N: w68 -> [_]
              shift-right: [w162] -> _
              shift-left: w67 -> [w162]
              shift-right: [w160] -> w64
              shift-left: w69 -> [w159]
              tunnel: w80 -> [w158]
              shift-right: [w155] -> _
              shift-left: w81 -> [w157]
              tunnel: w63 -> [w150]
              i -> [w154]
              n90 = Index Array(array=w162, index=w154) -> (element=w171:T20)
              n91 = Unbundle(w171) -> ("Points"=w170:i32[])  [unwired: 2 out]
              n92 = Array To Cluster(array=w170) -> (cluster=w169:T21)
              n93 = Unbundle(w169) -> ("Points[0]"=w149:i32, "Points[1]"=w146:i32, "Points[2]"=w161:i32, "Points[3]"=w167:i32)  [unwired: 5 out]
              n94 = Add(x=w149, y=10) -> (x+y=w147:i32)
              n95 = Subtract(x=w146, y=w167) -> (x-y=w166:i32)
              n96 = Subtract(x=w149, y=w161) -> (x-y=w168:i32)
              n97 = Square(x=w166) -> (x^2=w164:i32)
              n98 = Square(x=w168) -> (x^2=w165:i32)
              n99 = Add(x=w165, y=w164) -> (x+y=w163:i32)
              n100 = Square Root(x=w163) -> (sqrt(x)=w140:dbl)
              n101 = Multiply(x=w140, y=0.5) -> (x*y=w143:dbl)
              n102 = Add(x=w143, y=w146) -> (x+y=w145:dbl)
              n103 = Bundle(w147, w145) -> (w156:cluster{i32, dbl})  [unwired: 1 in]
              n104 = Multiply(x=w140, y=w158) -> (x*y=w153:dbl[])
              n105 = Index Array(array=w153) -> (element=w152:dbl)  [unwired: 1 in]
              n106 = Number To Fractional String(number=w152) -> (F-format string=w151:string)  [unwired: 3 in]
              n107 = call "IMAQ Overlay Text"("BG Color (Transparent)"=u32 0, "Text Color (black)"=u32 16448250, "Font, Size & Style"=w150, "String"=w151, "Origin"=w156, "Image"=w157) -> ("Image Out"=w155:T9)  [unwired: 4 in, 1 out]
              n108 = Build Array (concatenate)(w159, w153) -> (w160:dbl[])
            }
            n109 = local write "Distances"(w64) -> ()
            n110 = Add Array Elements(numeric array=w64) -> (sum=w65:dbl)
            n111 = local write "Total Width"(w65) -> ()
          }
        }
        n112 = Unbundle By Name(w52) -> ("Manual-Temp"=w57:bool, "Manual-Width"=w56:bool, "Manuel-Length"=w55:bool, "Manuel-Dielectric"=w54:bool, "Manual Comments"=w53:bool)
        n113 = stacked-sequence {
          tunnel: w57 -> [w483 _ _]
          tunnel: w56 -> [_ w493 _]
          tunnel: w55 -> [_ _ w508]
          tunnel: w54 -> [_ _ w505]
          tunnel: w53 -> [_ _ w504]
          frame #0 {
            n114 = local read "Rec: Temp"() -> (w482:dbl)
            n115 = case shown="False" w483 {
              tunnel: w482 -> [w488 _]
              tunnel: [w485 w492] -> _
              frame False {
                n116 = local read "Rec: Temp"() -> (w486:dbl)
                n117 = property on="New: Temp" class="DigNum (strict)"("DisabledEnum"=1) -> ()  [unwired: 2 in, 2 out]
                n118 = Equal To 0?(x=w486) -> (x = 0?=w487:bool)
                n119 = local write "New: Temp"(w488) -> ()
                n120 = case shown="True" w487 {
                  tunnel: [w489 w490] -> w485
                  tunnel: w486 -> [w489 _]
                  frame False {
                  }
                  frame True {
                    n121 = local read "Room Temp"() -> (w490:dbl)
                  }
                }
                n122 = local write "New: Temp"(w485) -> ()
              }
              frame True {
                n123 = property on="New: Temp" class="DigNum (strict)"("DisabledEnum"=0) -> ()  [unwired: 2 in, 2 out]
                n124 = local read "New: Temp"() -> (w492:dbl)
              }
            }
          }
          frame #1 {
            n125 = case shown="False" w493 {
              frame False {
                n126 = property on="New: Width" class="DigNum (strict)"("DisabledEnum"=1) -> ()  [unwired: 2 in, 2 out]
              }
              frame True {
                (unwired) 0
              }
            }
            n127 = local read "Total Width"() -> (w499:dbl)
            n128 = Equal To 0?(x=w499) -> (x = 0?=w496:bool)
            n129 = local read "Rec: Width"() -> (w497:dbl)
            n130 = Not(x=w493) -> (.not. x?=w495:bool)
            n131 = Or(x=w496, y=w493) -> (x .or. y?=w498:bool)
            n132 = And(x=w496, y=w495) -> (x .and. y?=w494:bool)
            n133 = case shown="True" w494 {
              tunnel: w497 -> [_ w501]
              frame False {
              }
              frame True {
                n134 = local write "New: Width"(w501) -> ()
              }
            }
            n135 = case shown="True" w498 {
              tunnel: w499 -> [w502 _]
              frame False {
                (unwired) 1
                n136 = local write "New: Width"(w502) -> ()
              }
              frame True {
                n137 = property on="New: Width" class="DigNum (strict)"("DisabledEnum"=0) -> ()  [unwired: 2 in, 2 out]
              }
            }
          }
          frame #2 {
            n138 = local read "Rec: Length"() -> (w509:dbl)
            n139 = case shown="True" w508 {
              tunnel: w509 -> [w517 _]
              frame False {
                n140 = local write "New: Length"(w517) -> ()
                n141 = property on="New: Length" class="DigNum (strict)"("DisabledEnum"=1) -> ()  [unwired: 2 in, 2 out]
              }
              frame True {
                n142 = property on="New: Length" class="DigNum (strict)"("DisabledEnum"=0) -> ()  [unwired: 2 in, 2 out]
              }
            }
            n143 = local read "Comments:"() -> (w506:string)
            n144 = local read "Rec: Dielectric (d)"() -> (w507:dbl)
            n145 = case shown="True" w504 {
              tunnel: w506 -> [w511 _]
              frame False {
                n146 = local write "New: Comments"(w511) -> ()
                n147 = property on="New: Comments" class="Str"("DisabledEnum"=1) -> ()  [unwired: 2 in, 2 out]
              }
              frame True {
                n148 = property on="New: Comments" class="Str"("DisabledEnum"=0) -> ()  [unwired: 2 in, 2 out]
              }
            }
            n149 = case shown="True" w505 {
              tunnel: w507 -> [w514 _]
              frame False {
                n150 = local write "New: Dielectric"(w514) -> ()
                n151 = property on="New: Dielectric" class="DigNum (strict)"("DisabledEnum"=1) -> ()  [unwired: 2 in, 2 out]
              }
              frame True {
                n152 = property on="New: Dielectric" class="DigNum (strict)"("DisabledEnum"=0) -> ()  [unwired: 2 in, 2 out]
              }
            }
          }
        }
        n153 = property on="Next File" class="Bool (strict)"("Value"=w47) -> (error out=w46:errorcluster)  [unwired: 2 in, 1 out]
        n154 = property on="Previous File" class="Bool (strict)"(error in=w46, "Value"=w47) -> (error out=w45:errorcluster)  [unwired: 1 in, 1 out]
        n155 = property on="Save" class="Bool (strict)"(error in=w45, "Value"=w47) -> (error out=w44:errorcluster)  [unwired: 1 in, 1 out]
        n156 = property on="Export" class="Bool (strict)"("Value"=w47) -> ()  [unwired: 2 in, 2 out]
        n157 = Unbundle By Name(w48) -> ()  [unwired: 8 out]
        n158 = property on="Save Next" class="Bool (strict)"(error in=w44, "Value"=w47) -> (error out=w43:errorcluster)  [unwired: 1 in, 1 out]
        n159 = property on="Discard" class="Bool (strict)"(error in=w43, "Value"=w47) -> (error out=w42:errorcluster)  [unwired: 1 in, 1 out]
        n160 = property on="Save Lines" class="Bool (strict)"(error in=w42, "Value"=w47) -> ()  [unwired: 1 in, 2 out]
        n161 = property on="Close" class="Bool (strict)"("Value"=w47) -> ()  [unwired: 2 in, 2 out]
        n162 = Cluster To Array(cluster=w48) -> (array=w59:bool[])
        n163 = call "Next State.vi"("Buttons []"=w59, "States []"=w60) -> ("Enum"=w51:T3)
        n164 = event shown="[8] \"Image Analysis \", \"1) Transport \": Value Change" {
          selector: _ -> [_ _ _ _ _ _ _ _ _ _ _]
          dyn-events: _ -> [_ _ _ _ _ _ _ _ _ _ _]
          timeout: 5 -> [_ _ _ _ _ _ _ _ _ _ _]
          tunnel: w51 -> [w390 _ _ _ _ _ _ _ _ _ _]
          tunnel: [w390 MegaAwesome_States."Re-Calculated Values" MegaAwesome_States."Re-Calculated Values" MegaAwesome_States."Re-Calculated Values" MegaAwesome_States."Re-Calculated Values" MegaAwesome_States."Calculated Values" MegaAwesome_States."Re-Calculated Values" MegaAwesome_States."Re-Calculated Values" MegaAwesome_States."Calculated Values" MegaAwesome_States."Re-Calculated Values" MegaAwesome_States."Re-Calculated Values"] -> w50
          event Timeout {
            n165 = event-data() -> ()  [unwired: 1 in, 2 out]
          }
          event "New: Dielectric": Value Change {
            n166 = event-data() -> ()  [unwired: 1 in, 5 out]
          }
          event "New: Length": Value Change {
            n167 = event-data() -> ()  [unwired: 1 in, 5 out]
          }
          event "New: Width": Value Change {
            n168 = event-data() -> ()  [unwired: 1 in, 5 out]
          }
          event "New: Temp": Value Change {
            n169 = event-data() -> ()  [unwired: 1 in, 5 out]
          }
          event "Num Pts Log", "Transport Style Controls", "Num Pts": Value Change {
            n170 = event-data() -> ()  [unwired: 1 in, 5 out]
          }
          event "Sat-Trans Slider": Value Change {
            n171 = event-data() -> ()  [unwired: 1 in, 5 out]
            n172 = local read "Sqrt-Sat"() -> (w419:cluster{dbl[], dbl[]}[])
            n173 = Decimate 1D Array(w419) -> (w403:cluster{dbl[], dbl[]}[], w404:cluster{dbl[], dbl[]}[])
            n174 = local read "Slider Min"() -> (w400:dbl)
            n175 = local read "Sat-Trans Slider"() -> (w398:dbl)
            n176 = Array To Cluster(array=w403) -> (cluster=w418:T22)
            n177 = local read "New: Dielectric"() -> (w413:dbl)
            n178 = local read "Num Pts"() -> (w396:dbl)
            n179 = local read "New: Width"() -> (w415:dbl)
            n180 = local read "New: Length"() -> (w414:dbl)
            n181 = Unbundle(w418) -> ("[0]"=w417:cluster{dbl[], dbl[]})  [unwired: 8 out]
            n182 = Absolute Value(x=w400) -> (abs(x)=w399:dbl)
            n183 = Unbundle(w417) -> (w401:dbl[], w416:dbl[])
            n184 = Add(x=w398, y=w399) -> (x+y=w397:dbl)
            n185 = Array Subset(array=w401, index=w397, length=w396) -> (w411:dbl[])
            n186 = local write "Sat Vg Array-Used"(w411) -> ()
            n187 = Array Subset(array=w416, index=w397, length=w396) -> (w412:dbl[])
            n188 = call "Mobility-Vt-Used Pts_Saturation.vi"("Width"=w415, "Length"=w414, "Dielectric (d)"=w413, "Sat Id Used"=w412, "Vg Used"=w411) -> ("Vt"=w407:dbl, "Mobility"=w408:dbl)  [unwired: 4 in, 1 out]
            n189 = local write "Index-Sat"(w397) -> ()
            n190 = local write "Sat Id-Used"(w412) -> ()
            n191 = Bundle(w411, w412) -> (w405:cluster{dbl[], dbl[]})  [unwired: 1 in]
            n192 = local read "Re-Calculated Values Cluster"() -> (w410:T10)
            n193 = Bundle By Name(cluster=w410, "Mobility-Sat"=w408, "Vt-Sat"=w407) -> (w409:T10)
            n194 = local write "Re-Calculated Values Cluster"(w409) -> ()
            n195 = Build Array (concatenate)(w403, w404, w405) -> (w402:cluster{dbl[], dbl[]}[])
            n196 = local write "Sqrt-Sat"(w402) -> ()
          }
          event "Lin-Trans Slider": Value Change {
            n197 = event-data() -> ()  [unwired: 1 in, 5 out]
            n198 = local read "Sqrt-Lin"() -> (w443:cluster{dbl[], dbl[]}[])
            n199 = Decimate 1D Array(w443) -> (w428:cluster{dbl[], dbl[]}[], w429:cluster{dbl[], dbl[]}[])
            n200 = local read "Slider Min"() -> (w425:dbl)
            n201 = Array To Cluster(array=w428) -> (cluster=w442:T22)
            n202 = local read "Lin-Trans Slider"() -> (w423:dbl)
            n203 = local read "New: Dielectric"() -> (w436:dbl)
            n204 = local read "Num Pts"() -> (w439:dbl)
            n205 = local read "New: Width"() -> (w438:dbl)
            n206 = local read "New: Length"() -> (w437:dbl)
            n207 = local read "Lin Vd"() -> (w420:dbl)
            n208 = Unbundle(w442) -> ("[0]"=w441:cluster{dbl[], dbl[]})  [unwired: 8 out]
            n209 = Absolute Value(x=w425) -> (abs(x)=w424:dbl)
            n210 = Unbundle(w441) -> (w426:dbl[], w440:dbl[])
            n211 = Add(x=w423, y=w424) -> (x+y=w422:dbl)
            n212 = Array Subset(array=w426, index=w422, length=w439) -> (w434:dbl[])
            n213 = local write "Lin-Vg Array-Used"(w434) -> ()
            n214 = Array Subset(array=w440, index=w422, length=w439) -> (w435:dbl[])
            n215 = call "Mobility-Vt-Used Pts_Linear.vi"("Width"=w438, "Length"=w437, "Vd"=w420, "Dielectric (d)"=w436, "Id Used"=w435, "Vg Used"=w434) -> ("Mobility"=w431:dbl)  [unwired: 3 in, 2 out]
            n216 = local write "Index-Lin"(w422) -> ()
            n217 = local write "Lin Id-Used"(w435) -> ()
            n218 = Bundle(w434, w435) -> (w430:cluster{dbl[], dbl[]})  [unwired: 1 in]
            n219 = local read "Re-Calculated Values Cluster"() -> (w433:T10)
            n220 = Bundle By Name(cluster=w433, "Moblitity-Lin"=w431) -> (w432:T10)
            n221 = local write "Re-Calculated Values Cluster"(w432) -> ()
            n222 = Build Array (concatenate)(w428, w429, w430) -> (w427:cluster{dbl[], dbl[]}[])
            n223 = local write "Sqrt-Lin"(w427) -> ()
          }
          event "Image Analysis", "1) Transport": Value Change {
            n224 = event-data() -> ()  [unwired: 1 in, 5 out]
          }
          event "Sat-Log Slider": Value Change {
            n225 = event-data() -> ()  [unwired: 1 in, 5 out]
            n226 = local read "Sat-Log"() -> (w447:cluster{dbl[], dbl[]}[])
            n227 = Decimate 1D Array(w447) -> (w454:cluster{dbl[], dbl[]}[], w455:cluster{dbl[], dbl[]}[])
            n228 = local read "Slider Min"() -> (w451:dbl)
            n229 = Array To Cluster(array=w454) -> (cluster=w464:T22)
            n230 = local read "Num Pts Log"() -> (w461:dbl)
            n231 = local read "Sat-Log Slider"() -> (w449:dbl)
            n232 = Unbundle(w464) -> ("[0]"=w463:cluster{dbl[], dbl[]})  [unwired: 8 out]
            n233 = Absolute Value(x=w451) -> (abs(x)=w450:dbl)
            n234 = Unbundle(w463) -> (w452:dbl[], w462:dbl[])
            n235 = Add(x=w449, y=w450) -> (x+y=w446:dbl)
            n236 = Array Subset(array=w452, index=w446, length=w461) -> (w459:dbl[])
            n237 = Array Subset(array=w462, index=w446, length=w461) -> (w460:dbl[])
            n238 = local write "Vg Array-Log-Used"(w459) -> ()
            n239 = local write "IndexLog-Sat"(w446) -> ()
            n240 = Bundle(w459, w460) -> (w445:cluster{dbl[], dbl[]})  [unwired: 1 in]
            n241 = call "STS-Used.vi"("Id Used"=w460, "Vg-Used"=w459) -> ("STS"=w456:dbl)  [unwired: 9 in]
            n242 = local write "Sat Id-Log-Used"(w460) -> ()
            n243 = local read "Re-Calculated Values Cluster"() -> (w458:T10)
            n244 = Bundle By Name(cluster=w458, "STS"=w456) -> (w457:T10)
            n245 = local write "Re-Calculated Values Cluster"(w457) -> ()
            n246 = Build Array (concatenate)(w454, w455, w445) -> (w453:cluster{dbl[], dbl[]}[])
            n247 = local write "Sat-Log"(w453) -> ()
          }
          event "Lin-Log Slider": Value Change {
            # "No Indicator for Lin-Log Slider Use"
            n248 = event-data() -> ()  [unwired: 1 in, 5 out]
            n249 = local read "Log-Lin"() -> (w468:cluster{dbl[], dbl[]}[])
            n250 = Decimate 1D Array(w468) -> (w474:cluster{dbl[], dbl[]}[], w475:cluster{dbl[], dbl[]}[])
            n251 = local read "Slider Min"() -> (w471:dbl)
            n252 = Array To Cluster(array=w474) -> (cluster=w481:T22)
            n253 = local read "Num Pts Log"() -> (w478:dbl)
            n254 = local read "Lin-Log Slider"() -> (w469:dbl)
            n255 = Unbundle(w481) -> ("[0]"=w480:cluster{dbl[], dbl[]})  [unwired: 8 out]
            n256 = Absolute Value(x=w471) -> (abs(x)=w470:dbl)
            n257 = Unbundle(w480) -> (w472:dbl[], w479:dbl[])
            n258 = Add(x=w469, y=w470) -> (x+y=w467:dbl)
            n259 = Array Subset(array=w472, index=w467, length=w478) -> (w476:dbl[])
            n260 = local write "Lin-Vg Array-Log Used"(w476) -> ()
            n261 = Array Subset(array=w479, index=w467, length=w478) -> (w477:dbl[])
            n262 = local write "IndexLog-Sat"(w467) -> ()
            n263 = Bundle(w476, w477) -> (w466:cluster{dbl[], dbl[]})  [unwired: 1 in]
            n264 = call "STS-Used.vi"("Id Used"=w477, "Vg-Used"=w476) -> ()  [unwired: 9 in, 1 out]
            n265 = local write "Lin Id-Log Used"(w477) -> ()
            n266 = Build Array (concatenate)(w474, w475, w466) -> (w473:cluster{dbl[], dbl[]}[])
            n267 = local write "Log-Lin"(w473) -> ()
          }
        }
      }
      frame "Read Data" {
        n268 = call "Recorded Values.vi"("Path"=w525) -> ("Recorded Char"=w543:T10, "Recorded Prop"=w533:T2, "Fabrication Prop"=w527:T5)  [unwired: 8 in]
        n269 = Strip Path(path=w525) -> (stripped path=w526:path, name=w524:string)
        n270 = local write "Fabrication Prop"(w527) -> ()
        n271 = local write "Recorded Prop"(w533) -> ()
        n272 = Unbundle By Name(w533) -> ("Date Recorded"=w532:string, "Index"=w530:string, "Length"=w531:dbl, "Width"=w529:dbl, "Sample Temp"=w528:dbl)
        n273 = local write "Recorded Values Cluster"(w543) -> ()
        n274 = Unbundle By Name(w533) -> ("Sample Temp"=w536:dbl)
        n275 = Unbundle By Name(w527) -> ("Dielectric (nm)"=w521:dbl, "Comments"=w520:string)
        n276 = List Folder(path=w526) -> (filenames=w522:string[])  [unwired: 3 in, 3 out]
        n277 = local write "Rec: Dielectric (d)"(w521) -> ()
        n278 = local write "Date Created"(w532) -> ()
        n279 = local write "Index"(w530) -> ()
        n280 = local write "Rec: Length"(w531) -> ()
        n281 = local write "Rec: Width"(w529) -> ()
        n282 = local write "Rec: Temp"(w528) -> ()
        n283 = Equal To 0?(x=w536) -> (x = 0?=w539:bool)
        n284 = Number To Decimal String(number=w536) -> (decimal integer string=w540:string)  [unwired: 1 in]
        n285 = local write "Comments:"(w520) -> ()
        n286 = Search 1D Array(1D array=w522, element=w524) -> (index of element=w519:i32)  [unwired: 1 in]
        n287 = Equal?(x="", y=w540) -> (x = y?=w538:bool)
        n288 = Index Array(array=w522, index=w519) -> (element=w523:string)
        n289 = Or(x=w539, y=w538) -> (x .or. y?=w537:bool)
        n290 = local write "Data Name:"(w523) -> ()
        n291 = case shown="False" w537 {
          tunnel: [w544 w545] -> w534
          tunnel: w536 -> [w544 _]
          frame False {
          }
          frame True {
            n292 = local read "Room Temp"() -> (w545:dbl)
          }
        }
        n293 = local write "New: Temp"(w534) -> ()
        n294 = Bundle By Name(cluster=w533, "Sample Temp"=w534) -> (w535:T2)
        n295 = local write "Recorded Prop"(w535) -> ()
      }
      frame "Calculated Values" {
        n296 = case shown="False" w549 {
          selector: w549 -> [w610 _]
          tunnel: w559 -> [w609 w620]
          tunnel: w547 -> [w608 w616]
          tunnel: w546 -> [w613 w614]
          frame False {
            n297 = call "TRF to TSP Plot_09_21_12a_JW.vi"("Plot Transport"=w610, "No Transport File"=w613, "Transport Folder"=w608, "Transfer File"=w609) -> ("Transport"=w611:cluster{ext[], ext[]}[], "Transport File"=w612:path)  [unwired: 5 in, 1 out]
            n298 = local write "Transport"(w611) -> ()
            n299 = local write "Transport\nFile"(w612) -> ()
          }
          frame True {
            n300 = local read "Transport Style Controls"() -> (w619:T11)
            n301 = call "TRF to TSP Plot_09_21_12a_JW.vi"("Transport Graph Properties"=w619, "No Transport File"=w614, "Transport Folder"=w616, "Transfer File"=w620) -> ("Transport"=w618:cluster{ext[], ext[]}[], "Transport File"=w615:path)  [unwired: 5 in, 1 out]
            n302 = Array Size(array=w618) -> (size(s)=w617:i32)
            n303 = local write "Transport"(w618) -> ()
            n304 = for {
              N: w617 -> [_]
              tunnel: w619 -> [w624]
              i -> [w623]
              n305 = Unbundle By Name(w624) -> ("Transport Line Size"=w621:u16, "Transport Line Color"=w622:u32)
              n306 = property on="Transport" class="XYGraph (strict)"("Active Plot"=w623, "Plot.Plot Color"=w622, "Plot.Line Width"=w621) -> ()  [unwired: 2 in, 2 out]
            }
            n307 = local write "Transport\nFile"(w615) -> ()
          }
        }
        n308 = case shown="True" w548 {
          tunnel: w579 -> [_ w607]
          tunnel: w578 -> [w600 w606]
          tunnel: w559 -> [_ w605]
          frame False {
            n309 = call "Vision Acquisition2"("Image Path"=w600) -> ("Image Out"=w599:T9)  [unwired: 25 in, 1 out]
            n310 = local write "Image Out"(w599) -> ()
            n311 = local write "Image Preview"(w599) -> ()
          }
          frame True {
            n312 = call "Image from TRF Display.vi"("No Image File"=w606, "Image Folder"=w607, "Transfer File"=w605) -> ("Image Preview"=w601:T9, "Image Out"=w602:T9, "Image File"=w603:path, "Image Name"=w604:string)  [unwired: 5 in]
            n313 = local write "Image File"(w603) -> ()
            n314 = local write "Image Name"(w604) -> ()
            n315 = local write "Image Out"(w602) -> ()
            n316 = local write "Image Preview"(w601) -> ()
          }
        }
        n317 = local read "Fabrication Prop"() -> (w588:T5)
        n318 = local read "Recorded Prop"() -> (w581:T2)
        n319 = local read "Calculated Values Cluster"() -> (w598:T10)
        n320 = call "Mobility-Vt Calculator-File.vi"("NumPts"=w583, "Path"=w559) -> ("Used Points"=w576:T23, "Graph Cluster"=w565:T24, "Lin Vd"=w572:dbl, "Output"=w596:T25)  [unwired: 6 in]
        n321 = call "STS Calculator-File.vi"("NumPts"=w582, "Path"=w559) -> ("Used Points"=w570:T26, "XY Graph-Sat"=w552:cluster{dbl[], dbl[]}[], "XY Graph-Lin"=w553:cluster{dbl[], dbl[]}[], "Ouput"=w591:cluster{"STS-Sat":dbl, "STS-Lin":dbl})  [unwired: 6 in]
        n322 = Unbundle By Name(w588) -> ("Dielectric (nm)"=w586:dbl)
        n323 = Unbundle By Name(w581) -> ("Sample Temp"=w580:dbl)
        n324 = Unbundle By Name(w596) -> ("Mobility-Sat"=w595:dbl, "Vt-Sat"=w587:dbl, "Mobility-Lin"=w594:dbl, "Off I-Sat"=w593:dbl, "On/Off I-Sat"=w592:dbl)  [unwired: 1 out]
        n325 = local write "Lin Vd"(w572) -> ()
        n326 = Unbundle By Name(w591) -> ("STS-Sat"=w585:dbl)  [unwired: 1 out]
        n327 = local write "Sat-Log"(w552) -> ()
        n328 = local write "Log-Lin"(w553) -> ()
        n329 = call "Trap Density_VT.vi"("VT"=w587, "Dielectric"=w586) -> ("Trap Density-VT"=w590:dbl)
        n330 = call "Trap Density_STS.vi"("Temp (T) [K]"=w580, "S.T.S. (S)"=w585, "Dielectric"=w586) -> ("Trap Density (N)"=w589:dbl)  [unwired: 8 in]
        n331 = Bundle By Name(cluster=w598, "Mobility-Sat"=w595, "Moblitity-Lin"=w594, "On/Off"=w592, "Off Current"=w593, "Vt-Sat"=w587, "STS"=w585, "Trap Density-VT"=w590, "Trap Density-STS"=w589) -> (w597:T10)
        n332 = Unbundle By Name(w570) -> ("Sat Vg Used"=w569:dbl[], "Sat Log(Id) Used"=w568:dbl[], "Lin Vg Used"=w567:dbl[], "Lin Log(Id) Used"=w566:dbl[], "STS Index-Sat"=w550:dbl, "STS Index-Lin"=w551:dbl)
        n333 = Unbundle By Name(w576) -> ("Sat Vg Used"=w575:dbl[], "Sat Sqrt(Id) Used"=w574:dbl[], "Lin Vg Used"=w573:dbl[], "Lin Sqrt(Id) Used"=w571:dbl[], "Index-Lin"=w561:dbl, "Index-Sat"=w560:dbl)
        n334 = local write "Vg Array-Log-Used"(w569) -> ()
        n335 = local write "Sat Id-Log-Used"(w568) -> ()
        n336 = local write "Lin-Vg Array-Log Used"(w567) -> ()
        n337 = local write "Lin Id-Log Used"(w566) -> ()
        n338 = local write "IndexLog-Sat"(w550) -> ()
        n339 = local write "Index-Lin"(w551) -> ()
        n340 = local write "Calculated Values Cluster"(w597) -> ()
        n341 = local write "Sat Vg Array-Used"(w575) -> ()
        n342 = local write "Sat Id-Used"(w574) -> ()
        n343 = local write "Lin-Vg Array-Used"(w573) -> ()
        n344 = local write "Lin Id-Used"(w571) -> ()
        n345 = local write "Index-Sat"(w560) -> ()
        n346 = local write "Index-Lin"(w561) -> ()
        n347 = local write "Lin-Log Slider"(w551) -> ()
        n348 = local write "Sat-Log Slider"(w550) -> ()
        n349 = local write "Sat-Trans Slider"(w560) -> ()
        n350 = local write "Lin-Trans Slider"(w561) -> ()
        n351 = Unbundle By Name(w565) -> ("Raw Sat"=w558:cluster{dbl[], dbl[]}[], "Sqrt Sat"=w562:cluster{dbl[], dbl[]}[], "Raw Lin"=w564:cluster{dbl[], dbl[]}[], "Sqrt Lin"=w563:cluster{dbl[], dbl[]}[])
        n352 = Index Array(array=w558) -> (element=w557:cluster{dbl[], dbl[]})  [unwired: 1 in]
        n353 = Unbundle(w557) -> (w556:dbl[])  [unwired: 1 out]
        n354 = Array Max & Min(array=w556) -> (max value=w555:dbl, min value=w554:dbl)  [unwired: 2 out]
        n355 = property on="Sat-Trans Slider" class="Slide (strict)"("Scale.Maximum"=w555, "Scale.Minimum"=w554) -> ()  [unwired: 2 in, 2 out]
        n356 = property on="Lin-Trans Slider" class="Slide (strict)"("Scale.Maximum"=w555, "Scale.Minimum"=w554) -> ()  [unwired: 2 in, 2 out]
        n357 = property on="Sat-Log Slider" class="Slide (strict)"("Scale.Maximum"=w555, "Scale.Minimum"=w554) -> ()  [unwired: 2 in, 2 out]
        n358 = property on="Lin-Log Slider" class="Slide (strict)"("Scale.Maximum"=w555, "Scale.Minimum"=w554) -> ()  [unwired: 2 in, 2 out]
        n359 = local write "Slider Max"(w555) -> ()
        n360 = local write "Slider Min"(w554) -> ()
        n361 = local write "Raw- Sat"(w558) -> ()
        n362 = local write "Raw- Lin"(w564) -> ()
        n363 = local write "Sqrt-Sat"(w562) -> ()
        n364 = local write "Sqrt-Lin"(w563) -> ()
      }
      frame "Re-Calculated Values" {
        n365 = local read "Vg Array-Log-Used"() -> (w633:dbl[])
        n366 = local read "Sat Vg Array-Used"() -> (w641:dbl[])
        n367 = local read "Lin-Vg Array-Used"() -> (w647:dbl[])
        n368 = local read "Sat Id-Log-Used"() -> (w632:dbl[])
        n369 = local read "New: Dielectric"() -> (w645:dbl)
        n370 = local read "New: Dielectric"() -> (w630:dbl)
        n371 = local read "New: Length"() -> (w644:dbl)
        n372 = local read "New: Length"() -> (w640:dbl)
        n373 = local read "New: Width"() -> (w643:dbl)
        n374 = local read "New: Width"() -> (w639:dbl)
        n375 = local read "Lin Id-Used"() -> (w646:dbl[])
        n376 = local read "Sat Id-Used"() -> (w638:dbl[])
        n377 = local read "Re-Calculated Values Cluster"() -> (w649:T10)
        n378 = local read "New: Dielectric"() -> (w629:dbl)
        n379 = local read "New: Temp"() -> (w628:dbl)
        n380 = local read "Lin Vd"() -> (w625:dbl)
        n381 = call "Mobility-Vt-Used Pts_Saturation.vi"("Width"=w639, "Length"=w640, "Dielectric (d)"=w630, "Sat Id Used"=w638, "Vg Used"=w641) -> ("Vt"=w636:dbl, "Mobility"=w637:dbl)  [unwired: 4 in, 1 out]
        n382 = call "STS-Used.vi"("Id Used"=w632, "Vg-Used"=w633) -> ("STS"=w631:dbl)  [unwired: 9 in]
        n383 = call "Mobility-Vt-Used Pts_Linear.vi"("Width"=w643, "Length"=w644, "Vd"=w625, "Dielectric (d)"=w645, "Id Used"=w646, "Vg Used"=w647) -> ("Mobility"=w642:dbl)  [unwired: 3 in, 2 out]
        n384 = call "Trap Density_VT.vi"("VT"=w636, "Dielectric"=w630) -> ("Trap Density-VT"=w635:dbl)
        n385 = call "Trap Density_STS.vi"("Temp (T) [K]"=w628, "S.T.S. (S)"=w631, "Dielectric"=w629) -> ("Trap Density (N)"=w627:dbl)  [unwired: 8 in]
        n386 = Bundle By Name(cluster=w649, "Mobility-Sat"=w637, "Moblitity-Lin"=w642, "Vt-Sat"=w636, "STS"=w631, "Trap Density-VT"=w635, "Trap Density-STS"=w627) -> (w648:T10)
        n387 = local write "Re-Calculated Values Cluster"(w648) -> ()
      }
      frame "Next File" {
        n388 = Strip Path(path=w666) -> (stripped path=w656:path, name=w664:string)
        n389 = local write "Transfer Folder"(w656) -> ()
        n390 = List Folder(path=w656) -> (filenames=w650:string[], error out=w659:errorcluster)  [unwired: 3 in, 2 out]
        n391 = Array Size(array=w650) -> (size(s)=w663:i32)
        n392 = Search 1D Array(1D array=w650, element=w664) -> (index of element=w661:i32)  [unwired: 1 in]
        n393 = Decrement(x=w663) -> (x-1=w662:i32)
        n394 = Equal?(x=w662, y=w661) -> (x = y?=w660:bool)
        n395 = case shown="False" w660 {
          tunnel: w652 -> [w669 _]
          tunnel: [w668 0] -> w651
          tunnel: w659 -> [w667 w670]
          tunnel: [w667 w670] -> _
          frame False {
            n396 = Increment(x=w669) -> (x+1=w668:i32)
          }
          frame True {
          }
        }
        n397 = Path To String(path=w656) -> (string=w657:string)
        n398 = Index Array(array=w650, index=w651) -> (element=w658:string)
        n399 = Concatenate Strings(w657, "\\", w658) -> (w654:string)
        n400 = String To Path(string=w654) -> (path=w653:path)
        n401 = local write "Transfer File"(w653) -> ()
      }
      frame "Previous File" {
        n402 = Strip Path(path=w678) -> (stripped path=w675:path, name=w687:string)
        n403 = local write "Transfer Folder"(w675) -> ()
        n404 = List Folder(path=w675) -> (filenames=w679:string[], error out=w684:errorcluster)  [unwired: 3 in, 2 out]
        n405 = Array Size(array=w679) -> (size(s)=w673:i32)
        n406 = Search 1D Array(1D array=w679, element=w687) -> (index of element=w686:i32)  [unwired: 1 in]
        n407 = Decrement(x=w673) -> (x-1=w672:i32)
        n408 = Equal To 0?(x=w686) -> (x = 0?=w685:bool)
        n409 = case shown="False" w685 {
          tunnel: w677 -> [w691 _]
          tunnel: [w690 w692] -> w676
          tunnel: w684 -> [w689 w693]
          tunnel: [w689 w693] -> _
          tunnel: w672 -> [_ w692]
          frame False {
            n410 = Decrement(x=w691) -> (x-1=w690:i32)
          }
          frame True {
          }
        }
        n411 = Path To String(path=w675) -> (string=w674:string)
        n412 = Index Array(array=w679, index=w676) -> (element=w683:string)
        n413 = Concatenate Strings(w674, "\\", w683) -> (w681:string)
        n414 = String To Path(string=w681) -> (path=w680:path)
        n415 = local write "Transfer File"(w680) -> ()
      }
      frame "Discard File" {
      }
      frame "Save" {
        n416 = stacked-sequence {
          seq-local: [w711 _] -> [_ w1208]
          seq-local: [w710 _] -> [_ w1206]
          tunnel: w702 -> [w712 w1209]
          frame #0 {
            # "Saves each Re-calculated parameter in sequence"
            n417 = stacked-sequence {
              tunnel: [_ _ _ _ _ _ _ _ _ _ _ _ _ w1176] -> w710
              tunnel: w712 -> [w732 _ _ _ _ _ _ _ _ _ _ _ _ _]
              frame #0 {
                n418 = call-poly <vilib>:"Read From Spreadsheet File.vi"("file path (dialog if empty)"=w732) -> ("all rows"=w731:string[][])  [unwired: 6 in, 4 out]
                n419 = Array Size(array=w731) -> (size(s)=w736:i32[])
                n420 = Array Subset(array=w731, index (row)=0, index (col)=0, length (col)=3) -> (w740:string[][])  [unwired: 1 in]
                n421 = Index Array(array=w736, index=0) -> (element=w734:i32)
                n422 = Reshape Array(w740, w734) -> (w733:string[])
                n423 = Search 1D Array(1D array=w733, element="Dielectric (nm):") -> (index of element=w743:i32)  [unwired: 1 in]
                n424 = Equal?(x=w743, y=-1) -> (x = y?=w742:bool)
                n425 = case shown="False" w742 {
                  tunnel: w731 -> [w751 w755]
                  tunnel: w743 -> [w747 _]
                  tunnel: [w746 w755] -> w741
                  frame False {
                    n426 = local read "Rec: Dielectric (d)"() -> (w753:dbl)
                    n427 = Number To Fractional String(number=w753) -> (F-format string=w748:string)  [unwired: 3 in]
                    n428 = Divide(x=w747, y=3) -> (x/y=w750:dbl)
                    n429 = To Word Integer(number=w750) -> (16bit integer=w749:i16)
                    n430 = Replace Array Subset(array=w751, new element=w748, index (row)=w749, index (col)=1) -> (w746:string[][])
                  }
                  frame True {
                  }
                }
                n431 = local write "Save Array"(w741) -> ()
              }
              frame #1 {
                n432 = local read "Save Array"() -> (w757:string[][])
                n433 = Array Size(array=w757) -> (size(s)=w760:i32[])
                n434 = Array Subset(array=w757, index (row)=0, index (col)=0, length (col)=3) -> (w764:string[][])  [unwired: 1 in]
                n435 = Index Array(array=w760, index=0) -> (element=w758:i32)
                n436 = Reshape Array(w764, w758) -> (w756:string[])
                n437 = Search 1D Array(1D array=w756, element="Comments:") -> (index of element=w767:i32)  [unwired: 1 in]
                n438 = Equal?(x=w767, y=-1) -> (x = y?=w766:bool)
                n439 = case shown="False" w766 {
                  tunnel: w757 -> [w775 w778]
                  tunnel: w767 -> [w772 _]
                  tunnel: [w771 w778] -> w765
                  frame False {
                    n440 = local read "New: Comments"() -> (w770:string)
                    n441 = Divide(x=w772, y=3) -> (x/y=w774:dbl)
                    n442 = To Word Integer(number=w774) -> (16bit integer=w773:i16)
                    n443 = Replace Array Subset(array=w775, new element=w770, index (row)=w773, index (col)=1) -> (w771:string[][])
                  }
                  frame True {
                  }
                }
                n444 = local write "Save Array"(w765) -> ()
              }
              frame #2 {
                n445 = local read "Save Array"() -> (w780:string[][])
                n446 = Array Size(array=w780) -> (size(s)=w783:i32[])
                n447 = Array Subset(array=w780, index (row)=0, index (col)=0, length (col)=3) -> (w787:string[][])  [unwired: 1 in]
                n448 = Index Array(array=w783, index=0) -> (element=w781:i32)
                n449 = Reshape Array(w787, w781) -> (w779:string[])
                n450 = Search 1D Array(1D array=w779, element="Length (um):") -> (index of element=w790:i32)  [unwired: 1 in]
                n451 = Equal?(x=w790, y=-1) -> (x = y?=w789:bool)
                n452 = case shown="False" w789 {
                  tunnel: w780 -> [w800 w803]
                  tunnel: w790 -> [w797 _]
                  tunnel: [w796 w803] -> w788
                  frame False {
                    n453 = local read "New: Length"() -> (w793:dbl)
                    n454 = Divide(x=w797, y=3) -> (x/y=w799:dbl)
                    n455 = Format Value(format string="%#g", value (0)=w793) -> (output string=w794:string)  [unwired: 1 in]
                    n456 = To Word Integer(number=w799) -> (16bit integer=w798:i16)
                    n457 = Replace Array Subset(array=w800, new element=w794, index (row)=w798, index (col)=1) -> (w796:string[][])
                  }
                  frame True {
                  }
                }
                n458 = local write "Save Array"(w788) -> ()
              }
              frame #3 {
                n459 = local read "Save Array"() -> (w805:string[][])
                n460 = Array Size(array=w805) -> (size(s)=w810:i32[])
                n461 = Array Subset(array=w805, index (row)=0, index (col)=0, length (col)=3) -> (w806:string[][])  [unwired: 1 in]
                n462 = Index Array(array=w810, index=0) -> (element=w812:i32)
                n463 = Reshape Array(w806, w812) -> (w804:string[])
                n464 = Search 1D Array(1D array=w804, element="Width (um):") -> (index of element=w815:i32)  [unwired: 1 in]
                n465 = Equal?(x=w815, y=-1) -> (x = y?=w814:bool)
                n466 = case shown="False" w814 {
                  tunnel: w815 -> [w823 _]
                  tunnel: w805 -> [w822 w828]
                  tunnel: [w821 w828] -> w813
                  frame False {
                    n467 = local read "New: Width"() -> (w818:dbl)
                    n468 = Divide(x=w823, y=3) -> (x/y=w825:dbl)
                    n469 = To Word Integer(number=w825) -> (16bit integer=w824:i16)
                    n470 = Format Value(format string="%#g", value (0)=w818) -> (output string=w819:string)  [unwired: 1 in]
                    n471 = Replace Array Subset(array=w822, new element=w819, index (row)=w824, index (col)=1) -> (w821:string[][])
                  }
                  frame True {
                  }
                }
                n472 = local write "Save Array"(w813) -> ()
              }
              frame #4 {
                w838 = "Sample Temp (K):"
                n473 = local read "Save Array"() -> (w830:string[][])
                n474 = Array Size(array=w830) -> (size(s)=w835:i32[])
                n475 = Array Subset(array=w830, index (row)=0, index (col)=0, length (col)=3) -> (w831:string[][])  [unwired: 1 in]
                n476 = Index Array(array=w835, index=0) -> (element=w837:i32)
                n477 = Reshape Array(w831, w837) -> (w829:string[])
                n478 = Search 1D Array(1D array=w829, element=w838) -> (index of element=w841:i32)  [unwired: 1 in]
                n479 = Equal?(x=w841, y=-1) -> (x = y?=w840:bool)
                n480 = case shown="False" w840 {
                  tunnel: w830 -> [w850 w864]
                  tunnel: w841 -> [w847 _]
                  tunnel: [w846 w863] -> w839
                  tunnel: w829 -> [_ w866]
                  tunnel: w838 -> [_ w853]
                  frame False {
                    n481 = local read "New: Temp"() -> (w844:dbl)
                    n482 = Divide(x=w847, y=3) -> (x/y=w849:dbl)
                    n483 = Format Value(format string="%#g", value (0)=w844) -> (output string=w843:string)  [unwired: 1 in]
                    n484 = To Word Integer(number=w849) -> (16bit integer=w848:i16)
                    n485 = Replace Array Subset(array=w850, new element=w843, index (row)=w848, index (col)=1) -> (w846:string[][])
                  }
                  frame True {
                    n486 = local read "New: Temp"() -> (w855:dbl)
                    n487 = Search 1D Array(1D array=w866, element="Width (um):") -> (index of element=w860:i32)  [unwired: 1 in]
                    n488 = Divide(x=w860, y=3) -> (x/y=w861:dbl)
                    n489 = To Word Integer(number=w861) -> (16bit integer=w859:i16)
                    n490 = Format Value(format string="%#g", value (0)=w855) -> (output string=w854:string)  [unwired: 1 in]
                    n491 = Build Array(w853, w854) -> (w857:string[])
                    n492 = Increment(x=w859) -> (x+1=w858:i16)
                    n493 = Insert Into Array(array=w864, index (row)=w858, new element=w857) -> (w863:string[][])  [unwired: 1 in]
                  }
                }
                n494 = local write "Save Array"(w839) -> ()
              }
              frame #5 {
                w876 = "Mobility-Sat (cm^2/Vs):"
                n495 = local read "Save Array"() -> (w868:string[][])
                n496 = Array Size(array=w868) -> (size(s)=w873:i32[])
                n497 = Array Subset(array=w868, index (row)=0, index (col)=0, length (col)=3) -> (w869:string[][])  [unwired: 1 in]
                n498 = Index Array(array=w873, index=0) -> (element=w875:i32)
                n499 = Reshape Array(w869, w875) -> (w867:string[])
                n500 = Search 1D Array(1D array=w867, element=w876) -> (index of element=w879:i32)  [unwired: 1 in]
                n501 = Equal?(x=w879, y=-1) -> (x = y?=w878:bool)
                n502 = case shown="False" w878 {
                  tunnel: w868 -> [w889 w899]
                  tunnel: w879 -> [w886 _]
                  tunnel: [w885 w898] -> w877
                  tunnel: w867 -> [_ w896]
                  tunnel: w876 -> [_ w894]
                  frame False {
                    n503 = local read "Re-Calculated Values Cluster"() -> (w882:T10)
                    n504 = Unbundle By Name(w882) -> ("Mobility-Sat"=w881:dbl)
                    n505 = Divide(x=w886, y=3) -> (x/y=w888:dbl)
                    n506 = To Word Integer(number=w888) -> (16bit integer=w887:i16)
                    n507 = Format Value(format string="%#g", value (0)=w881) -> (output string=w883:string)  [unwired: 1 in]
                    n508 = Replace Array Subset(array=w889, new element=w883, index (row)=w887, index (col)=1) -> (w885:string[][])
                  }
                  frame True {
                    n509 = local read "Re-Calculated Values Cluster"() -> (w893:T10)
                    n510 = Unbundle By Name(w893) -> ("Mobility-Sat"=w892:dbl)
                    n511 = Search 1D Array(1D array=w896, element="Mobility (cm^2/Vs):") -> (index of element=w902:i32)  [unwired: 1 in]
                    n512 = Divide(x=w902, y=3) -> (x/y=w903:dbl)
                    n513 = To Word Integer(number=w903) -> (16bit integer=w895:i16)
                    n514 = Format Value(format string="%#g", value (0)=w892) -> (output string=w897:string)  [unwired: 1 in]
                    n515 = Build Array(w894, w897) -> (w901:string[])
                    n516 = Replace Array Subset(array=w899, new element=w901, index (row)=w895) -> (w898:string[][])  [unwired: 1 in]
                  }
                }
                n517 = local write "Save Array"(w877) -> ()
              }
              frame #6 {
                w915 = "Mobility-Lin (cm^2/Vs):"
                n518 = local read "Save Array"() -> (w906:string[][])
                n519 = Array Size(array=w906) -> (size(s)=w912:i32[])
                n520 = Array Subset(array=w906, index (row)=0, index (col)=0, length (col)=3) -> (w908:string[][])  [unwired: 1 in]
                n521 = Index Array(array=w912, index=0) -> (element=w914:i32)
                n522 = Reshape Array(w908, w914) -> (w907:string[])
                n523 = Search 1D Array(1D array=w907, element=w915) -> (index of element=w918:i32)  [unwired: 1 in]
                n524 = Equal?(x=w918, y=-1) -> (x = y?=w917:bool)
                n525 = case shown="True" w917 {
                  tunnel: w906 -> [w928 w936]
                  tunnel: w918 -> [w925 _]
                  tunnel: [w924 w935] -> w916
                  tunnel: w907 -> [_ w934]
                  tunnel: w915 -> [_ w933]
                  frame False {
                    n526 = local read "Re-Calculated Values Cluster"() -> (w921:T10)
                    n527 = Unbundle By Name(w921) -> ("Moblitity-Lin"=w920:dbl)
                    n528 = Divide(x=w925, y=3) -> (x/y=w927:dbl)
                    n529 = To Word Integer(number=w927) -> (16bit integer=w926:i16)
                    n530 = Format Value(format string="%#g", value (0)=w920) -> (output string=w922:string)  [unwired: 1 in]
                    n531 = Replace Array Subset(array=w928, new element=w922, index (row)=w926, index (col)=1) -> (w924:string[][])
                  }
                  frame True {
                    n532 = local read "Re-Calculated Values Cluster"() -> (w932:T10)
                    n533 = Unbundle By Name(w932) -> ("Moblitity-Lin"=w931:dbl)
                    n534 = Search 1D Array(1D array=w934, element="Mobility-Sat (cm^2/Vs):") -> (index of element=w941:i32)  [unwired: 1 in]
                    n535 = Divide(x=w941, y=3) -> (x/y=w942:dbl)
                    n536 = To Word Integer(number=w942) -> (16bit integer=w940:i16)
                    n537 = Format Value(format string="%#g", value (0)=w931) -> (output string=w945:string)  [unwired: 1 in]
                    n538 = Build Array(w933, w945) -> (w938:string[])
                    n539 = Increment(x=w940) -> (x+1=w939:i16)
                    n540 = Insert Into Array(array=w936, index (row)=w939, new element=w938) -> (w935:string[][])  [unwired: 1 in]
                  }
                }
                n541 = local write "Save Array"(w916) -> ()
              }
              frame #7 {
                w955 = "On/Off I-Sat:"
                n542 = local read "Save Array"() -> (w946:string[][])
                n543 = Array Size(array=w946) -> (size(s)=w952:i32[])
                n544 = Array Subset(array=w946, index (row)=0, index (col)=0, length (col)=3) -> (w948:string[][])  [unwired: 1 in]
                n545 = Index Array(array=w952, index=0) -> (element=w954:i32)
                n546 = Reshape Array(w948, w954) -> (w947:string[])
                n547 = Search 1D Array(1D array=w947, element=w955) -> (index of element=w958:i32)  [unwired: 1 in]
                n548 = Equal?(x=w958, y=-1) -> (x = y?=w957:bool)
                n549 = case shown="True" w957 {
                  tunnel: w946 -> [w968 w977]
                  tunnel: w958 -> [w965 _]
                  tunnel: [w964 w978] -> w956
                  tunnel: w947 -> [_ w975]
                  tunnel: w955 -> [_ w973]
                  frame False {
                    n550 = local read "Re-Calculated Values Cluster"() -> (w961:T10)
                    n551 = Divide(x=w965, y=3) -> (x/y=w967:dbl)
                    n552 = Unbundle By Name(w961) -> ("On/Off"=w960:dbl)
                    n553 = To Word Integer(number=w967) -> (16bit integer=w966:i16)
                    n554 = Format Value(format string="%#g", value (0)=w960) -> (output string=w962:string)  [unwired: 1 in]
                    n555 = Replace Array Subset(array=w968, new element=w962, index (row)=w966, index (col)=1) -> (w964:string[][])
                  }
                  frame True {
                    n556 = local read "Re-Calculated Values Cluster"() -> (w972:T10)
                    n557 = Unbundle By Name(w972) -> ("On/Off"=w971:dbl)
                    n558 = Search 1D Array(1D array=w975, element="On/Off Current:") -> (index of element=w981:i32)  [unwired: 1 in]
                    n559 = Divide(x=w981, y=3) -> (x/y=w982:dbl)
                    n560 = To Word Integer(number=w982) -> (16bit integer=w974:i16)
                    n561 = Format Value(format string="%#g", value (0)=w971) -> (output string=w976:string)  [unwired: 1 in]
                    n562 = Build Array(w973, w976) -> (w980:string[])
                    n563 = Replace Array Subset(array=w977, new element=w980, index (row)=w974) -> (w978:string[][])  [unwired: 1 in]
                  }
                }
                n564 = local write "Save Array"(w956) -> ()
              }
              frame #8 {
                w994 = "Off I-Sat (A):"
                n565 = local read "Save Array"() -> (w985:string[][])
                n566 = Array Size(array=w985) -> (size(s)=w991:i32[])
                n567 = Array Subset(array=w985, index (row)=0, index (col)=0, length (col)=3) -> (w987:string[][])  [unwired: 1 in]
                n568 = Index Array(array=w991, index=0) -> (element=w993:i32)
                n569 = Reshape Array(w987, w993) -> (w986:string[])
                n570 = Search 1D Array(1D array=w986, element=w994) -> (index of element=w997:i32)  [unwired: 1 in]
                n571 = Equal?(x=w997, y=-1) -> (x = y?=w996:bool)
                n572 = case shown="True" w996 {
                  tunnel: w985 -> [w1007 w1015]
                  tunnel: w997 -> [w1004 _]
                  tunnel: [w1003 w1014] -> w995
                  tunnel: w986 -> [_ w1013]
                  tunnel: w994 -> [_ w1012]
                  frame False {
                    n573 = local read "Re-Calculated Values Cluster"() -> (w1000:T10)
                    n574 = Unbundle By Name(w1000) -> ("Off Current"=w999:dbl)
                    n575 = Divide(x=w1004, y=3) -> (x/y=w1006:dbl)
                    n576 = Format Value(format string="%#g", value (0)=w999) -> (output string=w1001:string)  [unwired: 1 in]
                    n577 = To Word Integer(number=w1006) -> (16bit integer=w1005:i16)
                    n578 = Replace Array Subset(array=w1007, new element=w1001, index (row)=w1005, index (col)=1) -> (w1003:string[][])
                  }
                  frame True {
                    n579 = local read "Re-Calculated Values Cluster"() -> (w1011:T10)
                    n580 = Unbundle By Name(w1011) -> ("Off Current"=w1010:dbl)
                    n581 = Search 1D Array(1D array=w1013, element="On/Off I-Sat:") -> (index of element=w1020:i32)  [unwired: 1 in]
                    n582 = Divide(x=w1020, y=3) -> (x/y=w1021:dbl)
                    n583 = To Word Integer(number=w1021) -> (16bit integer=w1019:i16)
                    n584 = Format Value(format string="%#g", value (0)=w1010) -> (output string=w1024:string)  [unwired: 1 in]
                    n585 = Build Array(w1012, w1024) -> (w1017:string[])
                    n586 = Increment(x=w1019) -> (x+1=w1018:i16)
                    n587 = Insert Into Array(array=w1015, index (row)=w1018, new element=w1017) -> (w1014:string[][])  [unwired: 1 in]
                  }
                }
                n588 = local write "Save Array"(w995) -> ()
              }
              frame #9 {
                w1026 = "Vt-Sat (V):"
                n589 = local read "Save Array"() -> (w1027:string[][])
                n590 = Array Size(array=w1027) -> (size(s)=w1032:i32[])
                n591 = Array Subset(array=w1027, index (row)=0, index (col)=0, length (col)=3) -> (w1028:string[][])  [unwired: 1 in]
                n592 = Index Array(array=w1032, index=0) -> (element=w1034:i32)
                n593 = Reshape Array(w1028, w1034) -> (w1025:string[])
                n594 = Search 1D Array(1D array=w1025, element=w1026) -> (index of element=w1037:i32)  [unwired: 1 in]
                n595 = Equal?(x=w1037, y=-1) -> (x = y?=w1036:bool)
                n596 = case shown="False" w1036 {
                  tunnel: w1027 -> [w1046 w1056]
                  tunnel: w1037 -> [w1042 _]
                  tunnel: [w1041 w1055] -> w1035
                  tunnel: w1026 -> [_ w1054]
                  tunnel: w1025 -> [_ w1053]
                  frame False {
                    n597 = local read "Re-Calculated Values Cluster"() -> (w1040:T10)
                    n598 = Unbundle By Name(w1040) -> ("Vt-Sat"=w1039:dbl)
                    n599 = Divide(x=w1042, y=3) -> (x/y=w1045:dbl)
                    n600 = To Word Integer(number=w1045) -> (16bit integer=w1044:i16)
                    n601 = Number To Fractional String(number=w1039) -> (F-format string=w1043:string)  [unwired: 3 in]
                    n602 = Replace Array Subset(array=w1046, new element=w1043, index (row)=w1044, index (col)=1) -> (w1041:string[][])
                  }
                  frame True {
                    n603 = local read "Re-Calculated Values Cluster"() -> (w1050:T10)
                    n604 = Unbundle By Name(w1050) -> ("Vt-Sat"=w1049:dbl)
                    n605 = Search 1D Array(1D array=w1053, element="Threshold V (V):") -> (index of element=w1052:i32)  [unwired: 1 in]
                    n606 = Divide(x=w1052, y=3) -> (x/y=w1059:dbl)
                    n607 = To Word Integer(number=w1059) -> (16bit integer=w1051:i16)
                    n608 = Format Value(format string="%#g", value (0)=w1049) -> (output string=w1062:string)  [unwired: 1 in]
                    n609 = Build Array(w1054, w1062) -> (w1058:string[])
                    n610 = Replace Array Subset(array=w1056, new element=w1058, index (row)=w1051) -> (w1055:string[][])  [unwired: 1 in]
                  }
                }
                n611 = local write "Save Array"(w1035) -> ()
              }
              frame #10 {
                n612 = disable-structure shown="Disabled" {
                  frame Disabled {
                    n613 = local read "Save Array"() -> (w1063:string[][])
                    n614 = Array Size(array=w1063) -> (size(s)=w1069:i32[])
                    n615 = Array Subset(array=w1063, index (row)=0, index (col)=0, length (col)=3) -> (w1065:string[][])  [unwired: 1 in]
                    n616 = Index Array(array=w1069, index=0) -> (element=w1071:i32)
                    n617 = Reshape Array(w1065, w1071) -> (w1064:string[])
                    n618 = Search 1D Array(1D array=w1064, element="VT-Lin (V):") -> (index of element=w1074:i32)  [unwired: 1 in]
                    n619 = Equal?(x=w1074, y=-1) -> (x = y?=w1073:bool)
                    n620 = case shown="False" w1073 {
                      tunnel: w1063 -> [w1083 w1086]
                      tunnel: w1074 -> [w1080 _]
                      tunnel: [w1079 w1086] -> w1072
                      frame False {
                        n621 = Divide(x=w1080, y=3) -> (x/y=w1082:dbl)
                        n622 = To Word Integer(number=w1082) -> (16bit integer=w1081:i16)
                        n623 = Format Value(format string="%#g") -> (output string=w1077:string)  [unwired: 2 in]
                        n624 = Replace Array Subset(array=w1083, new element=w1077, index (row)=w1081, index (col)=1) -> (w1079:string[][])
                      }
                      frame True {
                      }
                    }
                    n625 = local write "Save Array"(w1072) -> ()
                  }
                  frame Enabled {
                  }
                }
              }
              frame #11 {
                w1087 = "STS-Sat (V/decade):"
                n626 = local read "Save Array"() -> (w1089:string[][])
                n627 = Array Size(array=w1089) -> (size(s)=w1094:i32[])
                n628 = Array Subset(array=w1089, index (row)=0, index (col)=0, length (col)=3) -> (w1090:string[][])  [unwired: 1 in]
                n629 = Index Array(array=w1094, index=0) -> (element=w1096:i32)
                n630 = Reshape Array(w1090, w1096) -> (w1088:string[])
                n631 = Search 1D Array(1D array=w1088, element=w1087) -> (index of element=w1099:i32)  [unwired: 1 in]
                n632 = Equal?(x=w1099, y=-1) -> (x = y?=w1098:bool)
                n633 = case shown="True" w1098 {
                  tunnel: w1089 -> [w1109 w1117]
                  tunnel: w1099 -> [w1106 _]
                  tunnel: [w1105 w1118] -> w1097
                  tunnel: w1088 -> [_ w1116]
                  tunnel: w1087 -> [_ w1115]
                  frame False {
                    n634 = local read "Re-Calculated Values Cluster"() -> (w1101:T10)
                    n635 = Unbundle By Name(w1101) -> ("STS"=w1102:dbl)
                    n636 = Divide(x=w1106, y=3) -> (x/y=w1108:dbl)
                    n637 = To Word Integer(number=w1108) -> (16bit integer=w1107:i16)
                    n638 = Format Value(format string="%#g", value (0)=w1102) -> (output string=w1103:string)  [unwired: 1 in]
                    n639 = Replace Array Subset(array=w1109, new element=w1103, index (row)=w1107, index (col)=1) -> (w1105:string[][])
                  }
                  frame True {
                    n640 = local read "Re-Calculated Values Cluster"() -> (w1112:T10)
                    n641 = Unbundle By Name(w1112) -> ("STS"=w1113:dbl)
                    n642 = Search 1D Array(1D array=w1116, element="S.T.S. (V/decade):") -> (index of element=w1121:i32)  [unwired: 1 in]
                    n643 = Divide(x=w1121, y=3) -> (x/y=w1122:dbl)
                    n644 = To Word Integer(number=w1122) -> (16bit integer=w1114:i16)
                    n645 = Format Value(format string="%#g", value (0)=w1113) -> (output string=w1125:string)  [unwired: 1 in]
                    n646 = Build Array(w1115, w1125) -> (w1120:string[])
                    n647 = Replace Array Subset(array=w1117, new element=w1120, index (row)=w1114) -> (w1118:string[][])  [unwired: 1 in]
                  }
                }
                n648 = local write "Save Array"(w1097) -> ()
              }
              frame #12 {
                w1126 = "Trap Density-VT (Traps/Vcm^2):"
                n649 = local read "Save Array"() -> (w1128:string[][])
                n650 = Array Size(array=w1128) -> (size(s)=w1133:i32[])
                n651 = Array Subset(array=w1128, index (row)=0, index (col)=0, length (col)=3) -> (w1129:string[][])  [unwired: 1 in]
                n652 = Index Array(array=w1133, index=0) -> (element=w1135:i32)
                n653 = Reshape Array(w1129, w1135) -> (w1127:string[])
                n654 = Search 1D Array(1D array=w1127, element=w1126) -> (index of element=w1138:i32)  [unwired: 1 in]
                n655 = Equal?(x=w1138, y=-1) -> (x = y?=w1137:bool)
                n656 = case shown="True" w1137 {
                  tunnel: w1128 -> [w1148 w1155]
                  tunnel: w1138 -> [w1144 _]
                  tunnel: [w1143 w1156] -> w1136
                  tunnel: w1127 -> [_ w1154]
                  tunnel: w1126 -> [_ w1153]
                  frame False {
                    n657 = local read "Re-Calculated Values Cluster"() -> (w1141:T10)
                    n658 = Unbundle By Name(w1141) -> ("Trap Density-VT"=w1140:dbl)
                    n659 = Divide(x=w1144, y=3) -> (x/y=w1147:dbl)
                    n660 = To Word Integer(number=w1147) -> (16bit integer=w1146:i16)
                    n661 = Format Value(format string="%#g", value (0)=w1140) -> (output string=w1145:string)  [unwired: 1 in]
                    n662 = Replace Array Subset(array=w1148, new element=w1145, index (row)=w1146, index (col)=1) -> (w1143:string[][])
                  }
                  frame True {
                    n663 = local read "Re-Calculated Values Cluster"() -> (w1152:T10)
                    n664 = Unbundle By Name(w1152) -> ("Trap Density-VT"=w1151:dbl)
                    n665 = Search 1D Array(1D array=w1154, element="STS-Sat (V/decade):") -> (index of element=w1161:i32)  [unwired: 1 in]
                    n666 = Divide(x=w1161, y=3) -> (x/y=w1160:dbl)
                    n667 = To Word Integer(number=w1160) -> (16bit integer=w1162:i16)
                    n668 = Format Value(format string="%#g", value (0)=w1151) -> (output string=w1157:string)  [unwired: 1 in]
                    n669 = Build Array(w1153, w1157) -> (w1164:string[])
                    n670 = Increment(x=w1162) -> (x+1=w1163:i16)
                    n671 = Insert Into Array(array=w1155, index (row)=w1163, new element=w1164) -> (w1156:string[][])  [unwired: 1 in]
                  }
                }
                n672 = local write "Save Array"(w1136) -> ()
              }
              frame #13 {
                w1166 = "Trap Density-STS (Traps/Vcm^2):"
                n673 = local read "Save Array"() -> (w1168:string[][])
                n674 = Array Size(array=w1168) -> (size(s)=w1173:i32[])
                n675 = Array Subset(array=w1168, index (row)=0, index (col)=0, length (col)=3) -> (w1169:string[][])  [unwired: 1 in]
                n676 = Index Array(array=w1173, index=0) -> (element=w1175:i32)
                n677 = Reshape Array(w1169, w1175) -> (w1167:string[])
                n678 = Search 1D Array(1D array=w1167, element=w1166) -> (index of element=w1178:i32)  [unwired: 1 in]
                n679 = Equal?(x=w1178, y=-1) -> (x = y?=w1177:bool)
                n680 = case shown="True" w1177 {
                  tunnel: w1168 -> [w1188 w1195]
                  tunnel: w1178 -> [w1185 _]
                  tunnel: [w1184 w1196] -> w1176
                  tunnel: w1167 -> [_ w1194]
                  tunnel: w1166 -> [_ w1193]
                  frame False {
                    n681 = local read "Re-Calculated Values Cluster"() -> (w1181:T10)
                    n682 = Unbundle By Name(w1181) -> ("Trap Density-STS"=w1180:dbl)
                    n683 = Divide(x=w1185, y=3) -> (x/y=w1187:dbl)
                    n684 = To Word Integer(number=w1187) -> (16bit integer=w1186:i16)
                    n685 = Format Value(format string="%#g", value (0)=w1180) -> (output string=w1182:string)  [unwired: 1 in]
                    n686 = Replace Array Subset(array=w1188, new element=w1182, index (row)=w1186, index (col)=1) -> (w1184:string[][])
                  }
                  frame True {
                    n687 = local read "Re-Calculated Values Cluster"() -> (w1192:T10)
                    n688 = Unbundle By Name(w1192) -> ("Trap Density-STS"=w1191:dbl)
                    n689 = Search 1D Array(1D array=w1194, element="Trap Density-VT (Traps/Vcm^2):") -> (index of element=w1201:i32)  [unwired: 1 in]
                    n690 = Divide(x=w1201, y=3) -> (x/y=w1202:dbl)
                    n691 = To Word Integer(number=w1202) -> (16bit integer=w1200:i16)
                    n692 = Format Value(format string="%#g", value (0)=w1191) -> (output string=w1205:string)  [unwired: 1 in]
                    n693 = Build Array(w1193, w1205) -> (w1198:string[])
                    n694 = Increment(x=w1200) -> (x+1=w1199:i16)
                    n695 = Insert Into Array(array=w1195, index (row)=w1199, new element=w1198) -> (w1196:string[][])  [unwired: 1 in]
                  }
                }
                n696 = local write "Save Array"(w1176) -> ()
              }
            }
            n697 = local read "New: Temp"() -> (w713:dbl)
            n698 = local read "New: Width"() -> (w714:dbl)
            n699 = local read "New: Length"() -> (w716:dbl)
            n700 = local read "Index"() -> (w715:string)
            n701 = To Single Precision Float(number=w713) -> (single precision float=w730:sgl)
            n702 = Number To Decimal String(number=w730) -> (decimal integer string=w725:string)  [unwired: 1 in]
            n703 = To Single Precision Float(number=w714) -> (single precision float=w729:sgl)
            n704 = To Single Precision Float(number=w716) -> (single precision float=w728:sgl)
            n705 = Strip Path(path=w712) -> (stripped path=w717:path)  [unwired: 1 out]
            n706 = Number To Decimal String(number=w728) -> (decimal integer string=w723:string)  [unwired: 1 in]
            n707 = Number To Decimal String(number=w729) -> (decimal integer string=w722:string)  [unwired: 1 in]
            n708 = Concatenate Strings("_", w725, "K") -> (w727:string)
            n709 = call "Build Text"("Temp"=w727, "Index"=w715, "Length"=w723, "Width"=w722) -> ("Result"=w721:string)  [unwired: 10 in, 1 out]
            n710 = Path To String(path=w717) -> (string=w719:string)
            n711 = Concatenate Strings(w719, "\\", w721) -> (w720:string)
            n712 = String To Path(string=w720) -> (path=w711:path)
          }
          frame #1 {
            n713 = flat-sequence {
              tunnel: w1209 -> [w1211]
              tunnel: w1208 -> [w1210]
              tunnel: [w1210] -> w1207
              tunnel: w1207 -> [w1217]
              tunnel: w1206 -> [w1216]
              frame #0 {
                n714 = Equal?(x=w1211, y=w1210) -> (x = y?=w1212:bool)
                n715 = case shown="False" w1212 {
                  tunnel: w1211 -> [w1215 _]
                  tunnel: w1210 -> [w1214 _]
                  frame False {
                    n716 = Move(source path=w1215, 9:TRUE, 10:w1214) -> ()  [unwired: 2 in, 3 out]
                  }
                  frame True {
                  }
                }
              }
              frame #1 {
                n717 = local write "Transfer File"(w1217) -> ()
                n718 = call-poly <vilib>:"Write To Spreadsheet File.vi"("2D data"=w1216, "file path (dialog if empty)"=w1217) -> ()  [unwired: 6 in, 1 out]
              }
            }
          }
        }
        n719 = Cluster To Array(cluster=w701) -> (array=w700:bool[])
        n720 = Boolean Array To Number(Boolean array=w700) -> (number=w699:u32)
        n721 = Equal To 0?(x=w699) -> (x = 0?=w698:bool)
        n722 = case shown="True" w698 {
          tunnel: [MegaAwesome_States."Read Data" w705] -> w697
          tunnel: w696 -> [_ w709]
          frame False {
          }
          frame True {
            n723 = Unbundle By Name(w709) -> ("Save Next"=w708:bool)
            n724 = Select(t=MegaAwesome_States."No Event", s=w708, f=MegaAwesome_States."Next File") -> (s? t:f=w705:T3)
          }
        }
      }
      frame "Exit" {
      }
      frame "Save Lines" {
      }
      frame "Export" {
        n725 = flat-sequence {
          frame #0 {
            n726 = stacked-sequence {
              frame #0 {
                n727 = local read "Independant Variable:"() -> (w1224:string)
                n728 = Equal?(x=w1224, y="Length (um):") -> (x = y?=w1225:bool)
                n729 = case shown="True" w1225 {
                  frame False {
                  }
                  frame True {
                    n730 = local write "X Axis Display Type"("1") -> ()
                    n731 = local write "Opj X Axis"("2") -> ()
                  }
                }
              }
              frame #1 {
                n732 = local read "Independant Variable:"() -> (w1229:string)
                n733 = Equal?(x=w1229, y="Sample Temp (K):") -> (x = y?=w1230:bool)
                n734 = case shown="True" w1230 {
                  frame False {
                  }
                  frame True {
                    n735 = local write "X Axis Display Type"("1") -> ()
                    n736 = local write "Opj X Axis"("1") -> ()
                  }
                }
              }
              frame #2 {
                n737 = local read "Independant Variable:"() -> (w1234:string)
                n738 = Equal?(x=w1234, y="Mobility-Sat (cm^2/Vs):") -> (x = y?=w1235:bool)
                n739 = case shown="True" w1235 {
                  frame False {
                  }
                  frame True {
                    n740 = local write "X Axis Display Type"("2") -> ()
                    n741 = local write "Opj X Axis"("2") -> ()
                  }
                }
              }
              frame #3 {
                n742 = local read "Independant Variable:"() -> (w1239:string)
                n743 = Equal?(x=w1239, y="Mobility-Lin (cm^2/Vs):") -> (x = y?=w1240:bool)
                n744 = case shown="True" w1240 {
                  frame False {
                  }
                  frame True {
                    n745 = local write "X Axis Display Type"("2") -> ()
                    n746 = local write "Opj X Axis"("2") -> ()
                  }
                }
              }
              frame #4 {
                n747 = local read "Independant Variable:"() -> (w1244:string)
                n748 = Equal?(x=w1244, y="On/Off I-Sat:") -> (x = y?=w1245:bool)
                n749 = case shown="True" w1245 {
                  frame False {
                  }
                  frame True {
                    n750 = local write "X Axis Display Type"("2") -> ()
                    n751 = local write "Opj X Axis"("2") -> ()
                  }
                }
              }
              frame #5 {
                n752 = local read "Independant Variable:"() -> (w1249:string)
                n753 = Equal?(x=w1249, y="Off I-Sat (A):") -> (x = y?=w1250:bool)
                n754 = case shown="True" w1250 {
                  frame False {
                  }
                  frame True {
                    n755 = local write "X Axis Display Type"("2") -> ()
                    n756 = local write "Opj X Axis"("2") -> ()
                  }
                }
              }
              frame #6 {
                n757 = local read "Independant Variable:"() -> (w1254:string)
                n758 = Equal?(x=w1254, y="Vt-Sat (V):") -> (x = y?=w1255:bool)
                n759 = case shown="True" w1255 {
                  frame False {
                  }
                  frame True {
                    n760 = local write "X Axis Display Type"("1") -> ()
                    n761 = local write "Opj X Axis"("1") -> ()
                  }
                }
              }
              frame #7 {
                n762 = local read "Independant Variable:"() -> (w1259:string)
                n763 = Equal?(x=w1259, y="STS-Sat (V/decade):") -> (x = y?=w1260:bool)
                n764 = case shown="True" w1260 {
                  frame False {
                  }
                  frame True {
                    n765 = local write "X Axis Display Type"("1") -> ()
                    n766 = local write "Opj X Axis"("1") -> ()
                  }
                }
              }
              frame #8 {
                n767 = local read "Independant Variable:"() -> (w1264:string)
                n768 = Equal?(x=w1264, y="Trap Density-VT (Traps/Vcm^2):") -> (x = y?=w1265:bool)
                n769 = case shown="True" w1265 {
                  frame False {
                  }
                  frame True {
                    n770 = local write "X Axis Display Type"("2") -> ()
                    n771 = local write "Opj X Axis"("2") -> ()
                  }
                }
              }
              frame #9 {
                n772 = local read "Independant Variable:"() -> (w1269:string)
                n773 = Equal?(x=w1269, y="Trap Density-STS (Traps/Vcm^2):") -> (x = y?=w1270:bool)
                n774 = case shown="True" w1270 {
                  frame False {
                  }
                  frame True {
                    n775 = local write "X Axis Display Type"("2") -> ()
                    n776 = local write "Opj X Axis"("2") -> ()
                  }
                }
              }
            }
          }
          frame #1 {
            n777 = local read "Transfer Folder"() -> (w1278:path)
            n778 = Build Path(base path=w1278, name or relative path="Stats") -> (appended path=w1279:path)
            n779 = local read "Origin Project File"() -> (w1290:path)
            n780 = call <vilib>:"Check if File or Folder Exists.vi"("path"=w1279) -> ("file or folder exists?"=w1294:bool, "dup path"=w1293:path)  [unwired: 8 in, 1 out]
            n781 = call <userlib>:"OA_ConnectToOrigin.vi"() -> ("error out"=w1291:errorcluster, "Origin.IOApplication"=w1292:refnum<k7>)  [unwired: 8 in]
            n782 = case shown="False" w1294 {
              tunnel: w1293 -> [w1467 w1468]
              tunnel: [w1466 w1468] -> w1277
              frame False {
                n783 = Create Folder(path (use dialog)=w1467) -> (created path=w1466:path)  [unwired: 2 in, 2 out]
              }
              frame True {
              }
            }
            n784 = call "File Dialog"("start path"=w1279) -> ("selected path"=w1281:path)  [unwired: 11 in, 3 out]
            n785 = call <userlib>:"OA_Load.vi"("error in (no error)"=w1291, "Path"=w1290, "Origin.IOApplication"=w1292) -> ("error out"=w1288:errorcluster, "Origin.IOApplication"=w1289:refnum<k7>)  [unwired: 1 out]
            n786 = call "OAExecute.vi"("script"="document -m 3;", "Error IO"=w1288, "Origin.IOApplication"=w1289) -> ("Error IO Out"=w1286:errorcluster, "Origin.IOApplication"=w1287:refnum<k7>)  [unwired: 1 in, 1 out]
            n787 = local read "Independant Variable:"() -> (w1274:string)
            n788 = stacked-sequence {
              tunnel: w1278 -> [w1305 w1335 w1347 w1369 w1389 w1410 w1431 w1454]
              tunnel: w1277 -> [w1306 w1334 w1348 w1368 w1390 w1411 w1432 w1455]
              tunnel: w1287 -> [w1308 w1332 w1350 w1371 w1392 w1413 w1434 w1457]
              tunnel: w1286 -> [w1307 w1333 w1349 w1370 w1391 w1412 w1433 w1456]
              tunnel: [_ _ _ _ _ _ _ w1452] -> w1276
              tunnel: [_ _ _ _ _ _ _ w1453] -> w1275
              tunnel: w1274 -> [w1304 w1325 w1346 w1367 w1388 w1409 w1430 w1451]
              frame #0 {
                n789 = local read "X Axis Display Type"() -> (w1296:string)
                n790 = local read "Opj X Axis"() -> (w1301:string)
                n791 = Concatenate Strings("window -a MOBLGraph;\nlayer.x.type=", w1301, "; layer.x.label.numFormat = ", w1296, "; Y3 = 1; X3 = 1;", "window -a MOBLTable;\nwindow -s TV;") -> (w1299:string)
                n792 = call "Param_Analysis_7_24b_JW.vi"("Independant Variable"=w1304, "error in (no error)"=w1307, "Data Folder"=w1305, "Parameter String"="Mobility-Lin (cm^2/Vs):", "Parameter Name"="Mobility-Lin", "Stats Folder"=w1306) -> ("error out"=w1310:errorcluster, "Output Array"=w1312:string[][], "Variables"=w1303:T27)  [unwired: 2 in, 1 out]
                n793 = call "Origin_Export_7_27a_JW.vi"("Input Conditions"=w1303, "Analysis Array"=w1312, "error in (no error)"=w1310, "Parameter Worksheet Name"="[MOBLTable]Mobilities", "Parameter Folder Script"="pe_cd \"Mobility-Lin\";", "Origin.IOApplication"=w1308) -> ("error out"=w1309:errorcluster, "reference out"=w1311:refnum<k7>)  [unwired: 3 in, 1 out]
                n794 = call "OAExecute.vi"("script"=w1299, "Error IO"=w1309, "Origin.IOApplication"=w1311) -> ()  [unwired: 1 in, 3 out]
              }
              frame #1 {
                n795 = local read "X Axis Display Type"() -> (w1317:string)
                n796 = local read "Opj X Axis"() -> (w1322:string)
                n797 = Concatenate Strings("window -a MOBSGraph;\nlayer.x.type=", w1322, "; layer.x.label.numFormat = ", w1317, "; Y3 = 1; X3 = 1;", "window -a MOBSTable;\nwindow -s TV;") -> (w1320:string)
                n798 = call "Param_Analysis_7_24b_JW.vi"("Independant Variable"=w1325, "error in (no error)"=w1333, "Data Folder"=w1335, "Parameter String"="Mobility-Sat (cm^2/Vs):", "Parameter Name"="Mobility-Sat", "Stats Folder"=w1334) -> ("error out"=w1328:errorcluster, "Output Array"=w1326:string[][], "Variables"=w1324:T27)  [unwired: 2 in, 1 out]
                n799 = call "Origin_Export_7_27a_JW.vi"("Input Conditions"=w1324, "Analysis Array"=w1326, "error in (no error)"=w1328, "Parameter Worksheet Name"="[MOBSTable]Mobilities", "Parameter Folder Script"="pe_cd \"Mobility-Sat\";", "Origin.IOApplication"=w1332) -> ("error out"=w1327:errorcluster, "reference out"=w1329:refnum<k7>)  [unwired: 3 in, 1 out]
                n800 = call "OAExecute.vi"("script"=w1320, "Error IO"=w1327, "Origin.IOApplication"=w1329) -> ()  [unwired: 1 in, 3 out]
              }
              frame #2 {
                n801 = local read "X Axis Display Type"() -> (w1338:string)
                n802 = local read "Opj X Axis"() -> (w1343:string)
                n803 = Concatenate Strings("window -a NSTSGraph;\nlayer.x.type=", w1343, "; layer.x.label.numFormat = ", w1338, "; Y3 = 1; X3 = 1;", "window -a NSTSTable;\nwindow -s TV;") -> (w1341:string)
                n804 = call "Param_Analysis_7_24b_JW.vi"("Independant Variable"=w1346, "error in (no error)"=w1349, "Data Folder"=w1347, "Parameter String"="Trap Density-STS (Traps/Vcm^2):", "Parameter Name"="Trap Density-STS", "Stats Folder"=w1348) -> ("error out"=w1353:errorcluster, "Output Array"=w1351:string[][], "Variables"=w1345:T27)  [unwired: 2 in, 1 out]
                n805 = call "Origin_Export_7_27a_JW.vi"("Input Conditions"=w1345, "Analysis Array"=w1351, "error in (no error)"=w1353, "Parameter Worksheet Name"="[NSTSTable]Trap Densities", "Parameter Folder Script"="pe_cd \"N-STS\";", "Origin.IOApplication"=w1350) -> ("error out"=w1352:errorcluster, "reference out"=w1354:refnum<k7>)  [unwired: 3 in, 1 out]
                n806 = call "OAExecute.vi"("script"=w1341, "Error IO"=w1352, "Origin.IOApplication"=w1354) -> ()  [unwired: 1 in, 3 out]
              }
              frame #3 {
                n807 = local read "X Axis Display Type"() -> (w1359:string)
                n808 = local read "Opj X Axis"() -> (w1364:string)
                n809 = call "Param_Analysis_7_24b_JW.vi"("Independant Variable"=w1367, "error in (no error)"=w1370, "Data Folder"=w1369, "Parameter String"="Trap Density-VT (Traps/Vcm^2):", "Parameter Name"="Trap Density-Vt", "Stats Folder"=w1368) -> ("error out"=w1374:errorcluster, "Output Array"=w1372:string[][], "Variables"=w1366:T27)  [unwired: 2 in, 1 out]
                n810 = Concatenate Strings("window -a NVtGraph;\nlayer.x.type=", w1364, "; layer.x.label.numFormat = ", w1359, "; Y3 = 1; X3 = 1;", "window -a NVtTable;\nwindow -s TV;") -> (w1362:string)
                n811 = call "Origin_Export_7_27a_JW.vi"("Input Conditions"=w1366, "Analysis Array"=w1372, "error in (no error)"=w1374, "Parameter Worksheet Name"="[NVTTable]Trap Densities", "Parameter Folder Script"="pe_cd \"N-Vt\";", "Origin.IOApplication"=w1371) -> ("error out"=w1373:errorcluster, "reference out"=w1375:refnum<k7>)  [unwired: 3 in, 1 out]
                n812 = call "OAExecute.vi"("script"=w1362, "Error IO"=w1373, "Origin.IOApplication"=w1375) -> ()  [unwired: 1 in, 3 out]
              }
              frame #4 {
                n813 = local read "X Axis Display Type"() -> (w1380:string)
                n814 = local read "Opj X Axis"() -> (w1385:string)
                n815 = Concatenate Strings("window -a OffIGraph;\nlayer.x.type=", w1385, "; layer.x.label.numFormat = ", w1380, "; Y3 = 1; X3 = 1;", "window -a OffITable;\nwindow -s TV;") -> (w1383:string)
                n816 = call "Param_Analysis_7_24b_JW.vi"("Independant Variable"=w1388, "error in (no error)"=w1391, "Data Folder"=w1389, "Parameter String"="Off I-Sat (A):", "Parameter Name"="Off I-Sat", "Stats Folder"=w1390) -> ("error out"=w1395:errorcluster, "Output Array"=w1393:string[][], "Variables"=w1387:T27)  [unwired: 2 in, 1 out]
                n817 = call "Origin_Export_7_27a_JW.vi"("Input Conditions"=w1387, "Analysis Array"=w1393, "error in (no error)"=w1395, "Parameter Worksheet Name"="[OffItable]OffCurrents", "Parameter Folder Script"="pe_cd \"OffI-Sat\";", "Origin.IOApplication"=w1392) -> ("error out"=w1394:errorcluster, "reference out"=w1396:refnum<k7>)  [unwired: 3 in, 1 out]
                n818 = call "OAExecute.vi"("script"=w1383, "Error IO"=w1394, "Origin.IOApplication"=w1396) -> ()  [unwired: 1 in, 3 out]
              }
              frame #5 {
                n819 = local read "X Axis Display Type"() -> (w1401:string)
                n820 = local read "Opj X Axis"() -> (w1406:string)
                n821 = Concatenate Strings("window -a OnOffGraph;\nlayer.x.type=", w1406, "; layer.x.label.numFormat = ", w1401, "; Y3 = 1; X3 = 1;", "window -a OnOffTable;\nwindow -s TV;") -> (w1404:string)
                n822 = call "Param_Analysis_7_24b_JW.vi"("Independant Variable"=w1409, "error in (no error)"=w1412, "Data Folder"=w1410, "Parameter String"="On/Off I-Sat:", "Parameter Name"="OnOff Ratio", "Stats Folder"=w1411) -> ("error out"=w1416:errorcluster, "Output Array"=w1414:string[][], "Variables"=w1408:T27)  [unwired: 2 in, 1 out]
                n823 = call "Origin_Export_7_27a_JW.vi"("Input Conditions"=w1408, "Analysis Array"=w1414, "error in (no error)"=w1416, "Parameter Worksheet Name"="[OnOffTable]On/Off Ratios", "Parameter Folder Script"="pe_cd \"OnOff-Ratio\";", "Origin.IOApplication"=w1413) -> ("error out"=w1415:errorcluster, "reference out"=w1417:refnum<k7>)  [unwired: 3 in, 1 out]
                n824 = call "OAExecute.vi"("script"=w1404, "Error IO"=w1415, "Origin.IOApplication"=w1417) -> ()  [unwired: 1 in, 3 out]
              }
              frame #6 {
                n825 = local read "X Axis Display Type"() -> (w1422:string)
                n826 = local read "Opj X Axis"() -> (w1427:string)
                n827 = call "Param_Analysis_7_24b_JW.vi"("Independant Variable"=w1430, "error in (no error)"=w1433, "Data Folder"=w1431, "Parameter String"="STS-Sat (V/decade):", "Parameter Name"="STS-Sat", "Stats Folder"=w1432) -> ("error out"=w1437:errorcluster, "Output Array"=w1435:string[][], "Variables"=w1429:T27)  [unwired: 2 in, 1 out]
                n828 = Concatenate Strings("window -a SGraph;\nlayer.x.type=", w1427, "; layer.x.label.numFormat = ", w1422, "; Y3 = 1; X3 = 1;", "window -a STable;\nwindow -s TV;") -> (w1425:string)
                n829 = call "Origin_Export_7_27a_JW.vi"("Input Conditions"=w1429, "Analysis Array"=w1435, "error in (no error)"=w1437, "Parameter Worksheet Name"="[STable]Threshold Swing", "Parameter Folder Script"="pe_cd \"STS-Sat\";", "Origin.IOApplication"=w1434) -> ("error out"=w1436:errorcluster, "reference out"=w1438:refnum<k7>)  [unwired: 3 in, 1 out]
                n830 = call "OAExecute.vi"("script"=w1425, "Error IO"=w1436, "Origin.IOApplication"=w1438) -> ()  [unwired: 1 in, 3 out]
              }
              frame #7 {
                n831 = local read "X Axis Display Type"() -> (w1443:string)
                n832 = local read "Opj X Axis"() -> (w1448:string)
                n833 = Concatenate Strings("window -a VtGraph;\nlayer.x.type=", w1448, "; layer.x.label.numFormat = ", w1443, "; Y3 = 1; X3 = 1;", "window -a VtTable;\nwindow -s TV;") -> (w1446:string)
                n834 = call "Param_Analysis_7_24b_JW.vi"("Independant Variable"=w1451, "error in (no error)"=w1456, "Data Folder"=w1454, "Parameter String"="Vt-Sat (V):", "Parameter Name"="Vt-Sat", "Stats Folder"=w1455) -> ("error out"=w1460:errorcluster, "Output Array"=w1458:string[][], "Variables"=w1450:T27)  [unwired: 2 in, 1 out]
                n835 = call "Origin_Export_7_27a_JW.vi"("Input Conditions"=w1450, "Analysis Array"=w1458, "error in (no error)"=w1460, "Parameter Worksheet Name"="[VtTable]Threshold Voltages", "Parameter Folder Script"="pe_cd \"Vt-Sat\";", "Origin.IOApplication"=w1457) -> ("error out"=w1459:errorcluster, "reference out"=w1461:refnum<k7>)  [unwired: 3 in, 1 out]
                n836 = call "OAExecute.vi"("script"=w1446, "Error IO"=w1459, "Origin.IOApplication"=w1461) -> ("Error IO Out"=w1452:errorcluster, "Origin.IOApplication"=w1453:refnum<k7>)  [unwired: 1 in, 1 out]
              }
            }
            n837 = Path To String(path=w1281) -> (string=w1280:string)
            n838 = call "OAExecute.vi"("script"="pe_cd /; ", "Error IO"=w1276, "Origin.IOApplication"=w1275) -> ("Error IO Out"=w1282:errorcluster, "Origin.IOApplication"=w1283:refnum<k7>)  [unwired: 1 in, 1 out]
            n839 = call <userlib>:"OASaveProject.vi"("path"=w1280, "Error IO"=w1282, "Origin.IOApplication"=w1283) -> ()  [unwired: 3 out]
          }
        }
      }
    }
    "Current State" <- w19
    "Folder Index" <- w12
    n840 = Wait (ms)(milliseconds to wait=w6) -> ()  [unwired: 1 out]
    n841 = Equal?(x=w21, y=MegaAwesome_States."Exit") -> (x = y?=w22:bool)
  }
